vi "MegaAwesome_9_11_12a_JW.vi"() -> ()   [LabVIEW 2011]
uses:
  MegaAwesome_States.ctl
  <vilib>/Utility/inputDevices.llb/keyboardAcquire.vi
  <vilib>/Utility/file.llb/Read From Spreadsheet File (string).vi
  <vilib>/Utility/file.llb/Write To Spreadsheet File (string).vi
panel:
  in  "Slider Min":dbl=5.0
  in  "Slider Max":dbl=5.0
  out "Opj X Axis":string
  out "X Axis Display Type":string
  in  "Index-Sat":dbl=5.0
  in  "Index-Lin":dbl=5.0
  in  "IndexLog-Lin":dbl=5.0
  in  "IndexLog-Sat":dbl=5.0 caption="Num Pts"
  out "Lin Id-Log Used":dbl[](array[numeric])
  out "Lin-Vg Array-Log Used":dbl[](array[numeric])
  in  "New: Comments":string
  out "Save Array":string[][](array[string])
  out "Folder Index":i32 caption="Length"
  out "Sat Id-Used":dbl[](array[numeric])
  out "Sat Vg Array-Used":dbl[](array[numeric])
  out "Vg Array-Log-Used":dbl[](array[numeric])
  out "Sat Id-Log-Used":dbl[](array[numeric])
  out "Lin Id-Used":dbl[](array[numeric])
  out "Lin-Vg Array-Used":dbl[](array[numeric])
  out "Lin Vd":dbl
  out "Recorded Prop":T1
  out "Current State":T2
  in  "Main Tab Control":T3(tab)
  in  "Include Images?":bool
  in  "Image Folder":path
  out "Image File":path
  in  "Transfer File":path
  out "Transfer Folder":path
  out "Fabrication Prop":T4
  in  "Include Transport?":bool
  in  "Zoom":i16(slide)=-3 scale=-5.0..5.0
  in  "Magnification":u16(ring) items=["5x", "10x", "20x", "50x", "80x"]
  out "Distances":dbl[](array[numeric])
  in  "Undo Button":bool
  in  "Remove Button":bool
  in  "Transfer Plots":T5(tab)=enum."Saturation"
  in  "Lin-Trans Slider":dbl(slide) step=1.0 scale=-40.0..40.0 scale format="%#_1p"
  out "Sqrt-Lin":cluster{dbl[], dbl[]}[](graph)
  in  "Sat-Trans Slider":dbl(slide) step=1.0 scale=-40.0..40.0 scale format="%#_1p"
  out "Sqrt-Sat":cluster{dbl[], dbl[]}[](graph)
  out "Raw- Lin":cluster{dbl[], dbl[]}[](graph)
  out "Raw- Sat":cluster{dbl[], dbl[]}[](graph)
  in  "Log Plots":enum32{"Linear", "Saturation", "Transport"}(tab)=enum."Saturation"
  in  "Lin-Log Slider":dbl(slide) step=1.0 scale=-40.0..40.0 scale format="%#_1p"
  out "Log-Lin":cluster{dbl[], dbl[]}[](graph)
  in  "Sat-Log Slider":dbl(slide) step=1.0 scale=-40.0..40.0 scale format="%#_1p"
  out "Log-Sat":cluster{dbl[], dbl[]}[](graph)
  out "Transport":cluster{dbl[], dbl[]}[](graph)
  in  "Manual Controls":T6
  in  "File Controls":T7
  out "Date Recorded":string="Date Recorded" caption="Measured"
  out "Data Name:":string
  out "Image Name":string
  out "Index":string
  out "Date Created":string caption="Fabricated"
  in  "Comments:":string
  out "Rec: Length":dbl caption="Length" format="%#_3g"
  out "Rec: Width":dbl caption="Width" format="%#_4g"
  out "Rec: Dielectric (d)":dbl caption="Dielectric (d)" format="%#_3g"
  in  "New: Dielectric":dbl
  in  "New: Length":dbl
  in  "New: Width":dbl
  out "Rec: Temp":dbl caption="Sample Temp" format="%.1f"
  in  "New: Temp":dbl format="%.1f"
  out "Image Out":T8(plugin-control)
  in  "Num Pts":dbl=5.0
  in  "Num Pts Log":dbl=5.0 caption="Num Pts"
  out "Recorded Values Cluster":T9
  out "Calculated Values Cluster":T9 caption="Recorded Values Cluster"
  out "Re-Calculated Values Cluster":T9 caption="Recorded Values Cluster"
  in  "Independant Variable:":string(combo)="Length (um):"
  out "Image Preview":T8(plugin-control)
  out "Total Width":dbl
  in  "No Image File":path=path "\\\\acad1\\physics/Jurchescu-group/JW-PD/Mega Awesome/Image Not Found.png"
  in  "Room Temp":dbl=294.0
  in  "Origin Project File":path=path "\\\\acad1\\physics/Jurchescu-group/JW-PD/Group Library/Origin Project Files/DeviceData_8_10_12a_JW.opj"
  in  "Transport Style Controls":T10={"Transport Line Size"=1, "Transport Line Color"=16772608} {"Transport Line Size" items=["Extra Small", "Small", "Medium", "Large", "Extra Large"]}
  # "Image Location"
  # "(May not work with older versions)"
  # "Recorded"
  # "Calculated"
  # "Re-Calculated"
  # "Manual"
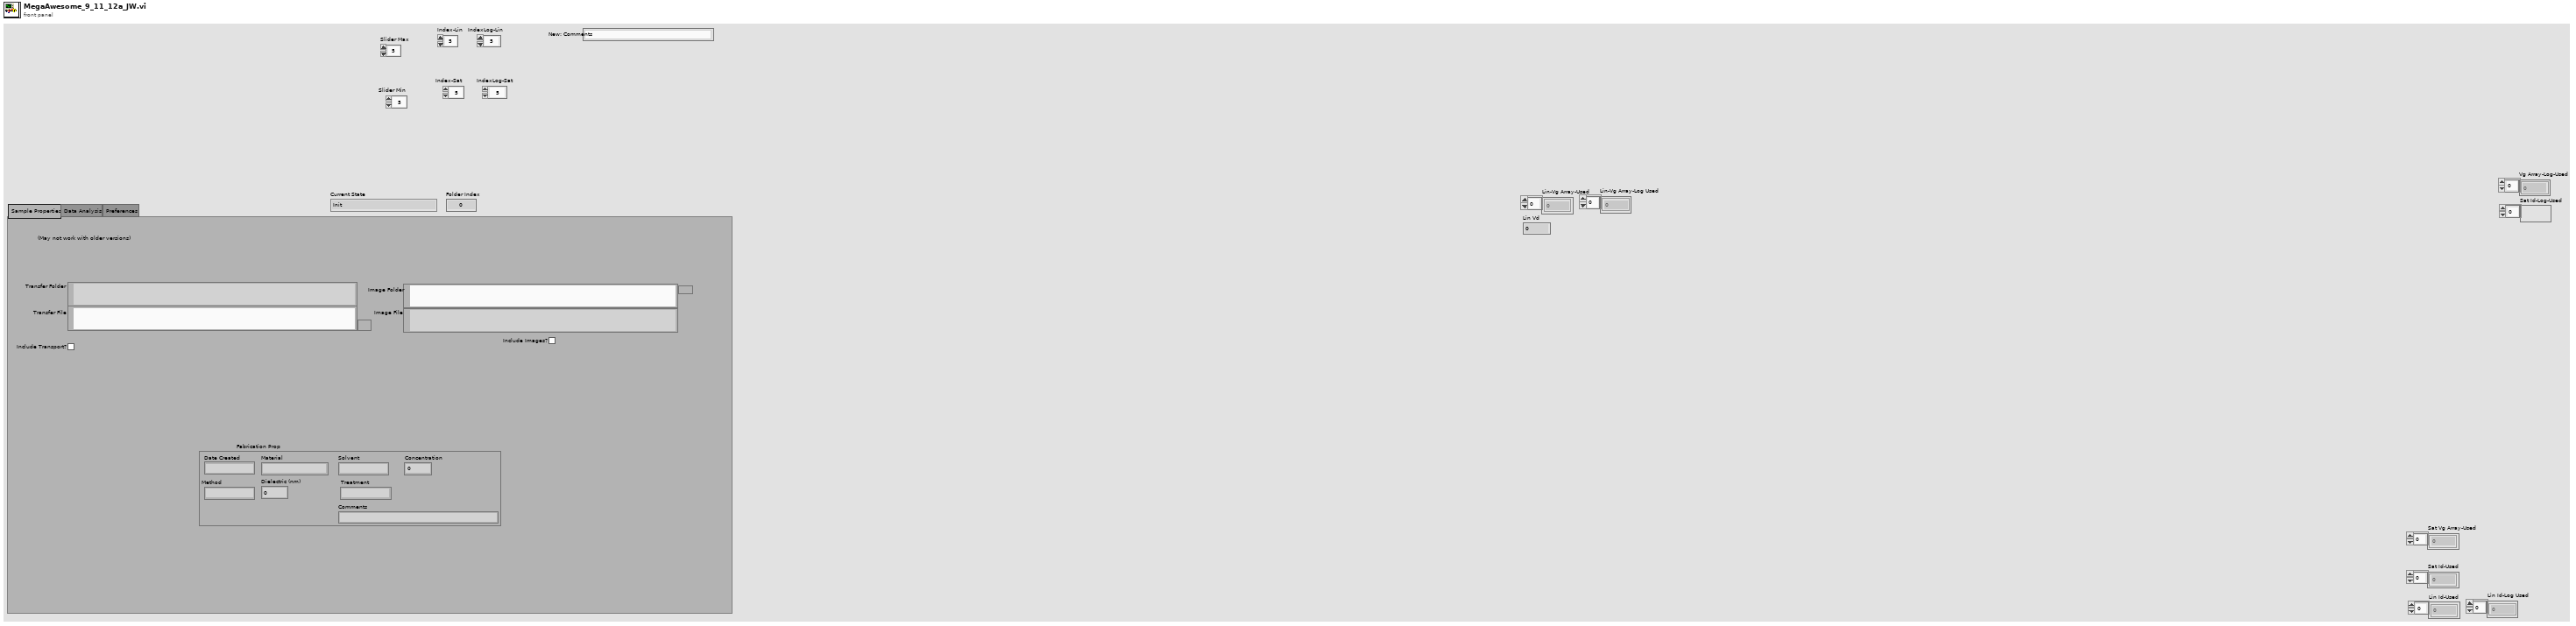
[diagram p1: front panel]
types:
  T1 = cluster{"Date Recorded":string, "Index":string, "Length":dbl, "Width":dbl, "Sample Temp":dbl}
  T2 = typedef "MegaAwesome_States.ctl" = enum16{"Init", "File Missing", "No Event", "Read Data", "Calculated Values", "Re-Calculated Values", "Next File", "Previous File", "Discard File", "Save", "Save Lines", "Export", "Exit"}
  T3 = enum32{"Sample Properties", "Data Analysis", "Preferences"}
  T4 = cluster{"Date Created":string, "Material":string, "Solvent":string, "Concentration":dbl, "Method":string, "Dielectric (nm)":dbl, "Treatment":string, "Comments":string}
  T5 = enum32{"Linear", "Saturation", "Raw-Linear", "Raw-Saturation"}
  T6 = cluster{"Manual-Temp":bool, "Manual-Width":bool, "Manuel-Length":bool, "Manuel-Dielectric":bool, "Manual Comments":bool}
  T7 = cluster{"Previous File":bool, "Discard ":bool, "Save Lines":bool, "Close":bool, "Next File ":bool, "Save":bool, "Save Next":bool, "Export":bool}
  T8 = typedef "IMAQ Image.ctl" = refnum<image>
  T9 = cluster{"Mobility-Sat":dbl, "Moblitity-Lin":dbl, "On/Off":dbl, "Off Current":dbl, "Vt-Sat":dbl, "STS":dbl, "Trap Density-VT":dbl, "Trap Density-STS":dbl}
  T10 = cluster{"Transport Line Size":u16, "Transport Line Color":u32}
  T11 = typedef "LVBoundsTypeDef.ctl" = cluster{"Width":u32, "Height":u32}
  T12 = cluster{"Global Rectangle":i32[], "Contours":cluster{"Contour Type":u32, "ROI Type":u32, "Points":i32[]}[]}
  T13 = cluster{"Contour Type":u32, "ROI Type":u32, "Points":i32[]}[]
  T14 = cluster{i32[], cluster{"Contour Type":u32, "ROI Type":u32, "Points":i32[]}[]}
  T15 = enum16{"0", "1", "2", "3", "4", "5", "6", "7", "8", "9", "A", "B", "C", "D", "E", "F", "G", "H", "I", "J", "K", "L", "M", "N", "O", "P", "Q", "R", "S", "T", "U", "V", "W", "X", "Y", "Z", "F1", "F2", "F3", "F4", "F5", "F6", "F7", "F8", "F9", "F10", "F11", "F12", "F13", "F14", "F15", "ADD", "BACK", "BACKSLASH", "CAPITAL", "COMMA", "DECIMAL", "DELETE", "DIVIDE", "DOWN", "END", "EQUALS", "ESCAPE", "GRAVE (`)", "HOME", "INSERT", "LBRACKET", "LCONTROL", "LEFT", "L ALT", "LSHIFT", "LWIN", "MINUS", "MULTIPLY", "NEXT", "NUMLOCK", "NUMPAD_0", "NUMPAD_1", "NUMPAD_2", "NUMPAD_3", "NUMPAD_4", "NUMPAD_5", "NUMPAD_6", "NUMPAD_7", "NUMPAD_8", "NUMPAD_9", "PAUSE", "PERIOD", "PRIOR (PG UP)", "RBRACKET", "RCONTROL", "RETURN", "RIGHT", "R ALT", "RSHIFT", "RWIN", "SCROLL", "SEMICOLON", "SLASH", "SPACE", "SUBTRACT", "TAB", "UP", "ENTER (num pad)", "' (quote)"}[]
  T16 = enum16{"0", "1", "2", "3", "4", "5", "6", "7", "8", "9", "A", "B", "C", "D", "E", "F", "G", "H", "I", "J", "K", "L", "M", "N", "O", "P", "Q", "R", "S", "T", "U", "V", "W", "X", "Y", "Z", "F1", "F2", "F3", "F4", "F5", "F6", "F7", "F8", "F9", "F10", "F11", "F12", "F13", "F14", "F15", "ADD", "BACK", "BACKSLASH", "CAPITAL", "COMMA", "DECIMAL", "DELETE", "DIVIDE", "DOWN", "END", "EQUALS", "ESCAPE", "GRAVE (`)", "HOME", "INSERT", "LBRACKET", "LCONTROL", "LEFT", "L ALT", "LSHIFT", "LWIN", "MINUS", "MULTIPLY", "NEXT", "NUMLOCK", "NUMPAD_0", "NUMPAD_1", "NUMPAD_2", "NUMPAD_3", "NUMPAD_4", "NUMPAD_5", "NUMPAD_6", "NUMPAD_7", "NUMPAD_8", "NUMPAD_9", "PAUSE", "PERIOD", "PRIOR (PG UP)", "RBRACKET", "RCONTROL", "RETURN", "RIGHT", "R ALT", "RSHIFT", "RWIN", "SCROLL", "SEMICOLON", "SLASH", "SPACE", "SUBTRACT", "TAB", "UP", "ENTER (num pad)", "' (quote)"}
  T17 = typedef "ROI Descriptor" = cluster{"Global Rectangle":i32[], "Contours":cluster{"ID":enum32{"External", "Internal"}, "Type":u32, "Coordinates":i32[]}[]}
  T18 = cluster{string, sgl, bool, bool, bool, bool, bool, bool, i32}
  T19 = cluster{i32, cluster{string, sgl, bool, bool, bool, bool, bool, bool, i32}, i32, i32}
  T20 = cluster{"Contour Type":u32, "ROI Type":u32, "Points":i32[]}
  T21 = cluster{"Points[0]":i32, "Points[1]":i32, "Points[2]":i32, "Points[3]":i32, "Points[4]":i32, "Points[5]":i32, "Points[6]":i32, "Points[7]":i32, "Points[8]":i32}
  T22 = cluster{"[0]":cluster{dbl[], dbl[]}, "[1]":cluster{dbl[], dbl[]}, "[2]":cluster{dbl[], dbl[]}, "[3]":cluster{dbl[], dbl[]}, "[4]":cluster{dbl[], dbl[]}, "[5]":cluster{dbl[], dbl[]}, "[6]":cluster{dbl[], dbl[]}, "[7]":cluster{dbl[], dbl[]}, "[8]":cluster{dbl[], dbl[]}}
  T23 = cluster{"Sat Vg Used":dbl[], "Sat Sqrt(Id) Used ":dbl[], "Lin Vg Used":dbl[], "Lin Sqrt(Id) Used":dbl[], "Index-Lin":dbl, "Index-Sat":dbl}
  T24 = cluster{"Raw Sat":cluster{dbl[], dbl[]}[], "Sqrt Sat":cluster{dbl[], dbl[]}[], "Log Sat":cluster{dbl[], dbl[]}[], "Raw Lin":cluster{dbl[], dbl[]}[], "Sqrt Lin":cluster{dbl[], dbl[]}[], "Log Lin":cluster{dbl[], dbl[]}[]}
  T25 = cluster{"Mobility-Sat":dbl, "Vt-Sat":dbl, "Mobility-Lin":dbl, "Vt-Lin":dbl, "Off I-Sat":dbl, "On/Off I-Sat":dbl}
  T26 = cluster{"Sat Vg Used":dbl[], "Sat Log(Id) Used":dbl[], "Lin Vg Used":dbl[], "Lin Log(Id) Used":dbl[], "STS Index-Sat":dbl, "STS Index-Lin":dbl}
  T27 = cluster{"Independant  Variable Indicator":string, "Parameter String Indicator":string}
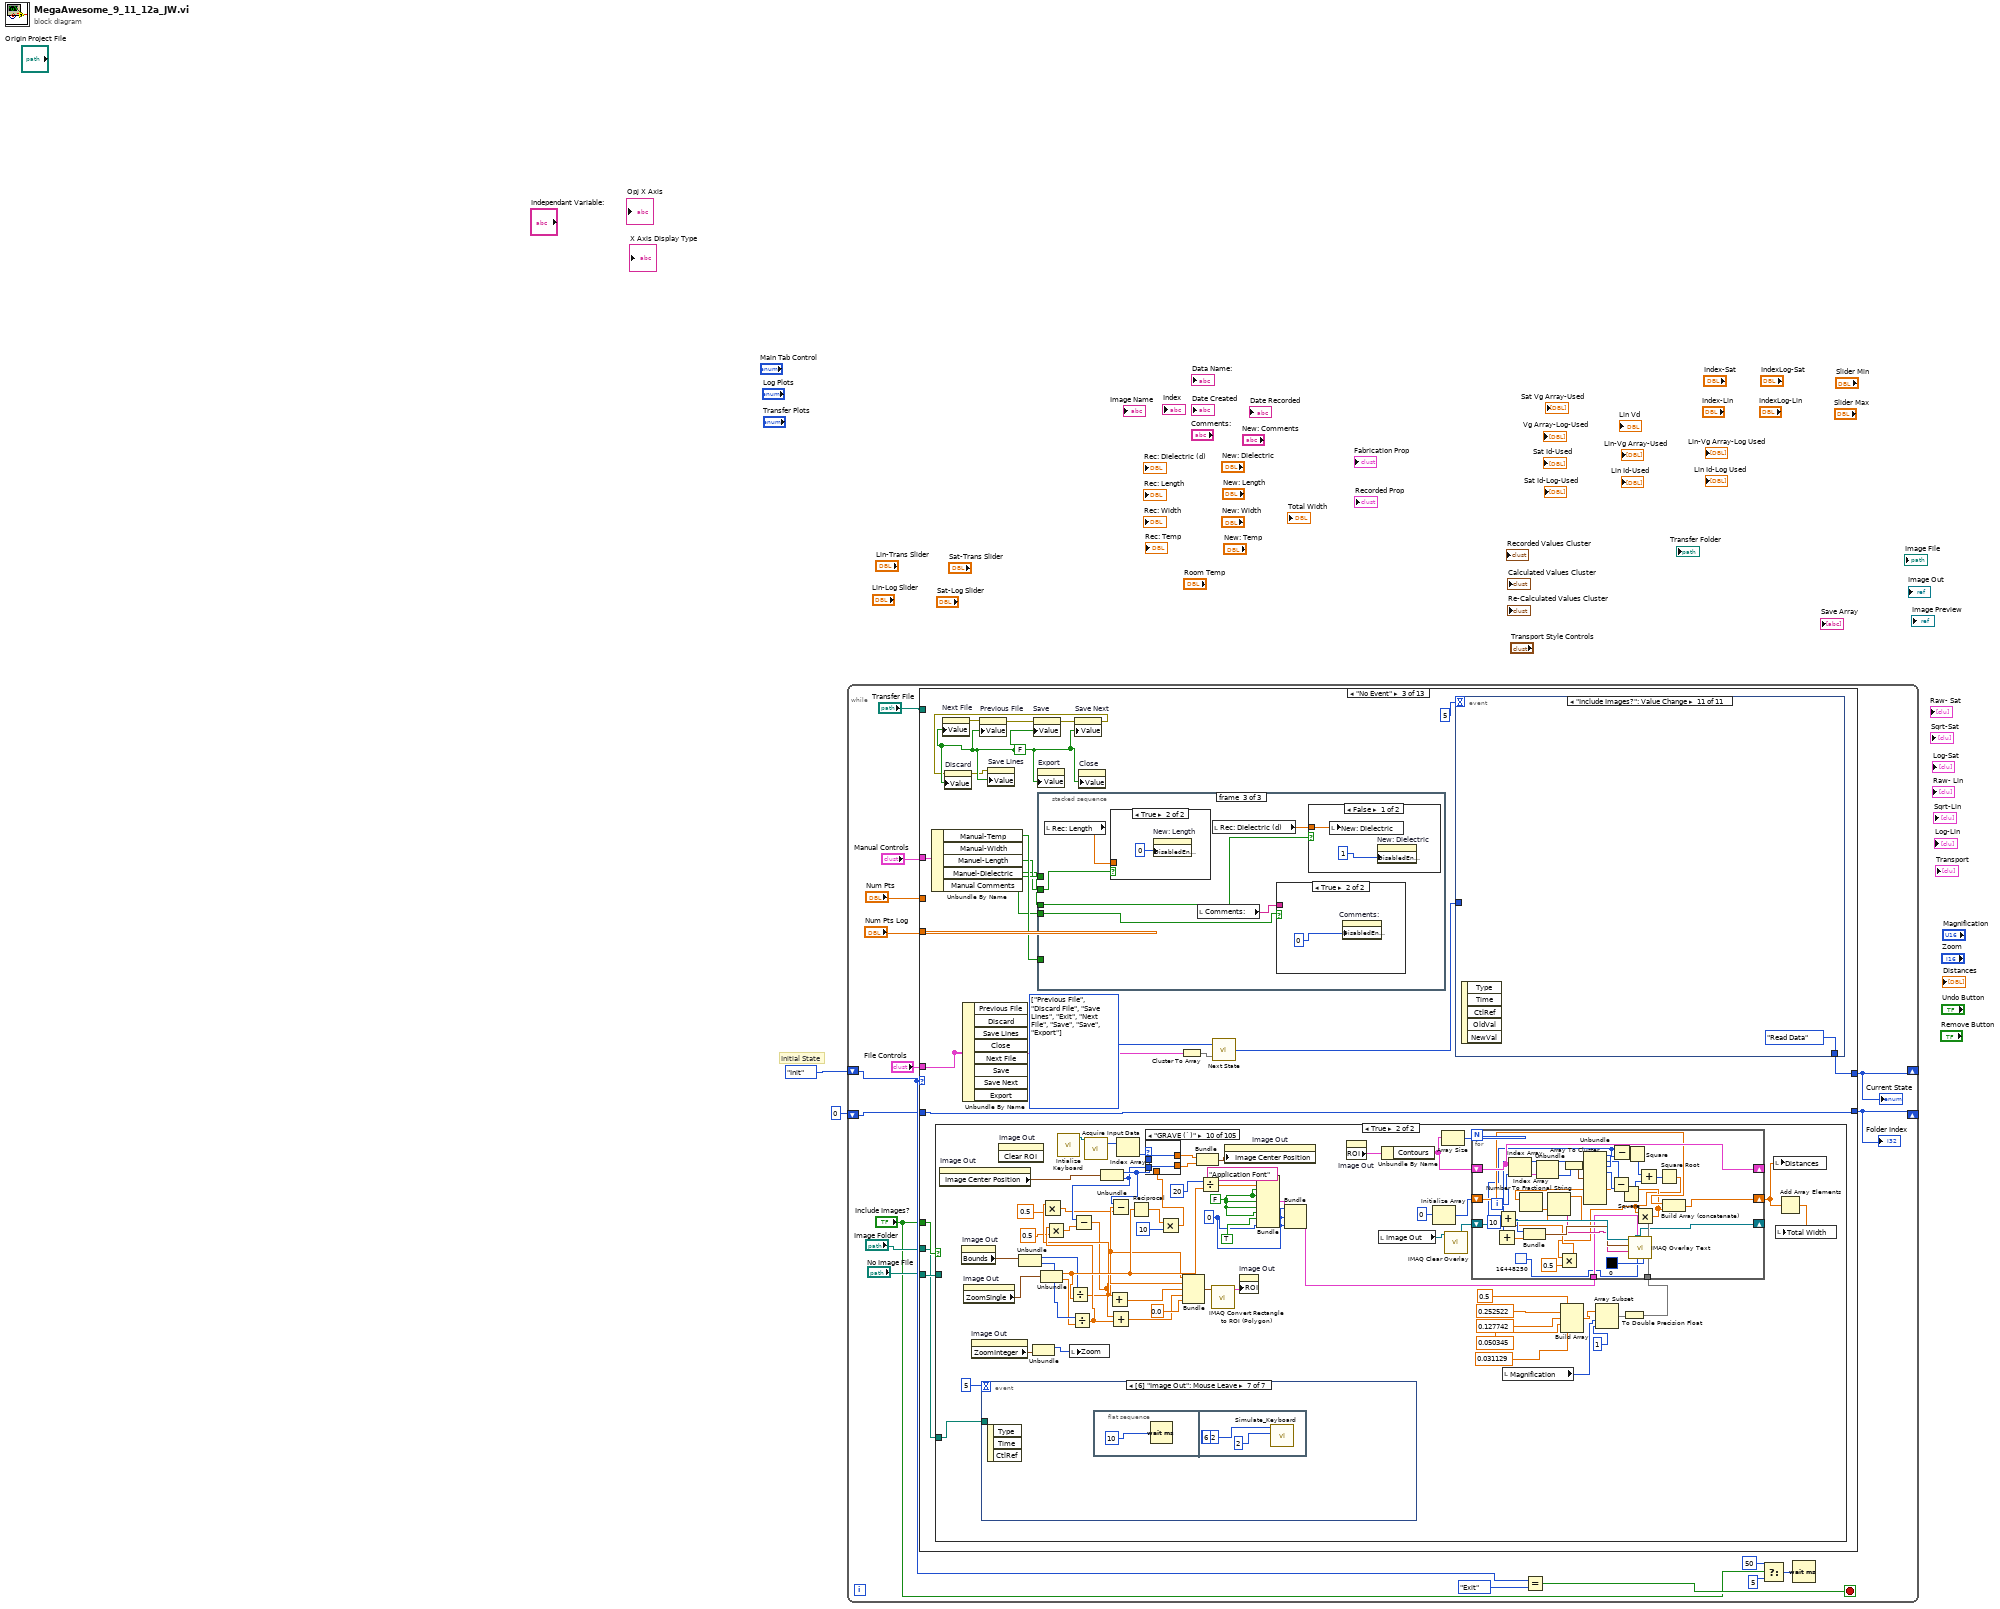
[diagram p0: block diagram]
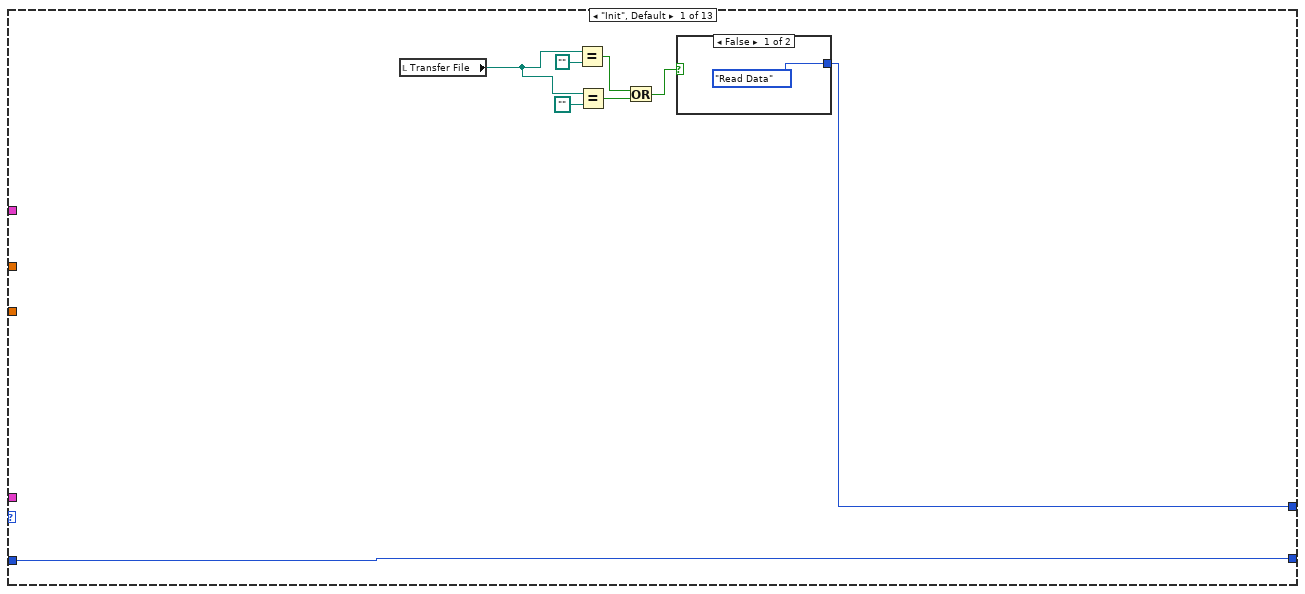
[diagram p2: hidden frame]
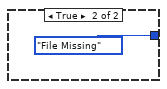
[diagram p3: hidden frame]
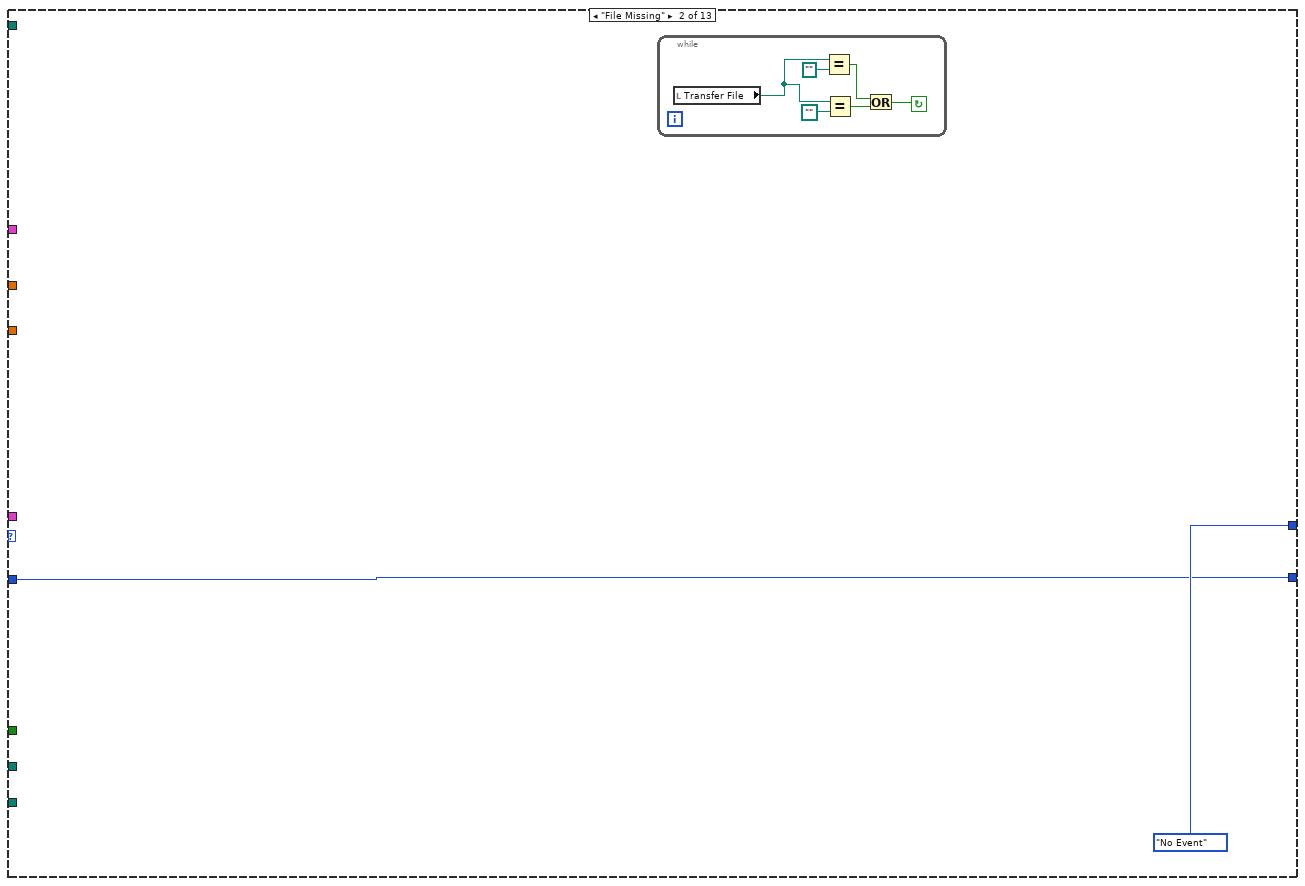
[diagram p4: hidden frame]
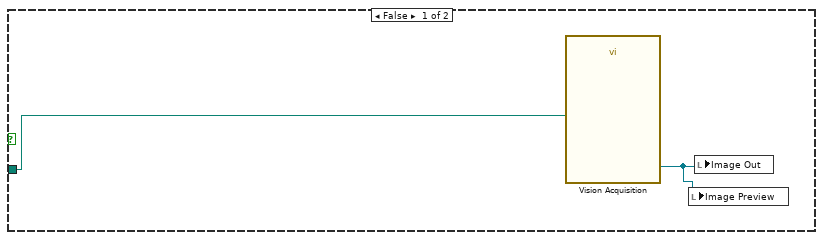
[diagram p5: hidden frame]
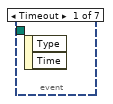
[diagram p6: hidden frame]
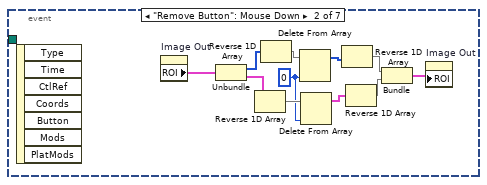
[diagram p7: hidden frame]
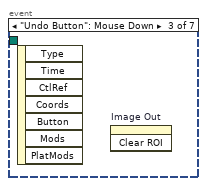
[diagram p8: hidden frame]
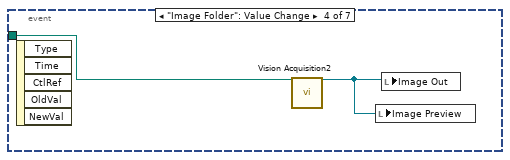
[diagram p9: hidden frame]
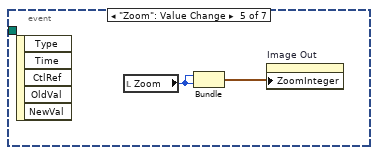
[diagram p10: hidden frame]
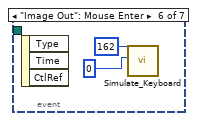
[diagram p11: hidden frame]
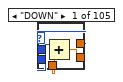
[diagram p12: hidden frame]
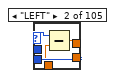
[diagram p13: hidden frame]
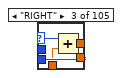
[diagram p14: hidden frame]
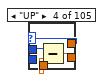
[diagram p15: hidden frame]
diagram:
  # "Initial State"
  n1 = while {
    shift-right: [w16] -> _
    shift-left: MegaAwesome_States."Init" -> [w18]
    shift-right: [w9] -> _
    shift-left: 0 -> [w10]
    stop <- w19 stop-if-true
    n2 = case shown="\"No Event\"" w18 {
      tunnel: [w21 MegaAwesome_States."No Event" w49 MegaAwesome_States."Calculated Values" MegaAwesome_States."Re-Calculated Values" MegaAwesome_States."No Event" MegaAwesome_States."Read Data" MegaAwesome_States."Read Data" MegaAwesome_States."No Event" w688 MegaAwesome_States."No Event" MegaAwesome_States."No Event" MegaAwesome_States."Exit"] -> w16
      tunnel: "Transfer File" -> [_ _ _ w529 w561 _ w657 w669 _ w693 _ _ _]
      tunnel: "Num Pts" -> [_ _ _ _ w585 _ _ _ _ _ _ _ _]
      tunnel: "Num Pts Log" -> [_ _ _ _ w584 _ _ _ _ _ _ _ _]
      tunnel: "Image Folder" -> [_ _ w38 _ w581 _ _ _ _ _ _ w1213 _]
      tunnel: "No Image File" -> [_ _ w39 _ w580 _ _ _ _ _ _ _ _]
      tunnel: [w20 w30 w57 w523 w579 w617 w642 w667 w685 w694 w1209 w1222 w1226] -> w9
      tunnel: w10 -> [w20 w30 w57 _ w579 w617 w643 w668 w685 w694 w1209 w1222 w1226]
      tunnel: "Manual Controls" -> [_ _ w51 _ _ _ _ _ _ w692 _ _ _]
      tunnel: "File Controls" -> [_ _ w47 _ _ _ _ _ _ w687 _ _ _]
      tunnel: "Include Images?" -> [_ _ w40 _ w550 _ _ _ _ _ _ _ _]
      frame "Init", Default {
        n3 = local read "Transfer File"() -> (w22:path)
        n4 = Equal?(x=w22, y=path "") -> (x = y?=w25:bool)
        n5 = Equal?(x=w22, y=path "") -> (x = y?=w24:bool)
        n6 = Or(x=w25, y=w24) -> (x .or. y?=w27:bool)
        n7 = case shown="False" w27 {
          tunnel: [MegaAwesome_States."Read Data" MegaAwesome_States."File Missing"] -> w21
          frame False {
          }
          frame True {
          }
        }
      }
      frame "File Missing" {
        n8 = while {
          stop <- w32 continue-if-true
          n9 = local read "Transfer File"() -> (w33:path)
          n10 = Equal?(x=w33, y=path "") -> (x = y?=w35:bool)
          n11 = Equal?(x=w33, y=path "") -> (x = y?=w36:bool)
          n12 = Or(x=w35, y=w36) -> (x .or. y?=w32:bool)
        }
      }
      frame "No Event" {
        w46 = FALSE
        w59 = T2[] [enum."Previous File", enum."Discard File", enum."Save Lines", enum."Exit", enum."Next File", enum."Save", enum."Save", enum."Export"] items=["Init", "File Missing", "No Event", "Read Data", "Calculated Values", "Re-Calculated Values", "Next File", "Previous File", "Discard File", "Save", "Save Lines", "Export", "Exit"]
        n13 = Unbundle By Name(w51) -> ("Manual-Temp"=w56:bool, "Manual-Width"=w55:bool, "Manuel-Length"=w54:bool, "Manuel-Dielectric"=w53:bool, "Manual Comments"=w52:bool)
        n14 = case shown="True" w40 {
          tunnel: w39 -> [w60 _]
          tunnel: w38 -> [_ w62]
          frame False {
            n15 = call "Vision Acquisition"("Image Path"=w60) -> ("Image Out"=w61:T8)  [unwired: 25 in, 1 out]
            n16 = local write "Image Preview"(w61) -> ()
            n17 = local write "Image Out"(w61) -> ()
          }
          frame True {
            w114 = FALSE
            w116 = 0
            n18 = property on="Image Out" class="ImageControl"() -> ("Image Center Position"=w86:cluster{"X":u32, "Y":u32})  [unwired: 2 in, 2 out]
            n19 = property on="Image Out" class="ImageControl"() -> ("Bounds"=w87:T11)  [unwired: 2 in, 2 out]
            n20 = property on="Image Out" class="ImageControl"() -> ("ZoomSingle"=w88:cluster{"X":sgl, "Y":sgl})  [unwired: 2 in, 2 out]
            n21 = property on="Image Out" class="ImageControl"() -> ("ZoomInteger"=w89:cluster{"X":i32, "Y":i32})  [unwired: 2 in, 2 out]
            n22 = event shown="[6] \"Image Out\": Mouse Leave" {
              selector: _ -> [_ _ _ _ _ _ _]
              dyn-events: _ -> [_ _ _ _ _ _ _]
              timeout: 5 -> [_ _ _ _ _ _ _]
              tunnel: w62 -> [_ _ _ w136 _ _ _]
              event Timeout {
                n23 = event-data() -> ()  [unwired: 1 in, 2 out]
              }
              event "Remove Button": Mouse Down {
                w124 = 0
                n24 = event-data() -> ()  [unwired: 1 in, 7 out]
                n25 = property on="Image Out" class="ImageControl"() -> ("ROI"=w126:T12)  [unwired: 2 in, 2 out]
                n26 = Unbundle(w126) -> ("Global Rectangle"=w134:i32[], "Contours"=w132:T13)
                n27 = Reverse 1D Array(array=w132) -> (reversed array=w131:T13)
                n28 = Reverse 1D Array(array=w134) -> (reversed array=w133:i32[])
                n29 = Delete From Array(array=w133, index=w124) -> (array with subset deleted=w130:i32[])  [unwired: 1 in, 1 out]
                n30 = Delete From Array(array=w131, index=w124) -> (array with subset deleted=w129:T13)  [unwired: 1 in, 1 out]
                n31 = Reverse 1D Array(array=w130) -> (reversed array=w128:i32[])
                n32 = Reverse 1D Array(array=w129) -> (reversed array=w127:T13)
                n33 = Bundle(w128, w127) -> (w125:T14)  [unwired: 1 in]
                n34 = property on="Image Out" class="ImageControl"("ROI"=w125) -> ()  [unwired: 2 in, 2 out]
              }
              event "Undo Button": Mouse Down {
                n35 = event-data() -> ()  [unwired: 1 in, 7 out]
                n36 = invoke on="Image Out" class="ImageControl" method="Clear ROI"() -> ()  [unwired: 3 in, 3 out]
              }
              event "Image Folder": Value Change {
                n37 = event-data() -> ()  [unwired: 1 in, 5 out]
                n38 = call "Vision Acquisition2"("Image Path"=w136) -> ("Image Out"=w135:T8)  [unwired: 25 in, 1 out]
                n39 = local write "Image Preview"(w135) -> ()
                n40 = local write "Image Out"(w135) -> ()
              }
              event "Zoom": Value Change {
                n41 = event-data() -> ()  [unwired: 1 in, 5 out]
                n42 = local read "Zoom"() -> (w138:i16)
                n43 = Bundle("Zoom"=w138, "Zoom"=w138) -> (w137:cluster{"Zoom":i16, "Zoom":i16})  [unwired: 1 in]
                n44 = property on="Image Out" class="ImageControl"("ZoomInteger"=w137) -> ()  [unwired: 2 in, 2 out]
              }
              event "Image Out": Mouse Enter {
                n45 = event-data() -> ()  [unwired: 1 in, 3 out]
                n46 = call "Simulate_Keyboard.vi"("Action"=0, "Virtual Key"=162) -> ()  [unwired: 7 in, 1 out]
              }
              event "Image Out": Mouse Leave {
                n47 = event-data() -> ()  [unwired: 1 in, 3 out]
                n48 = flat-sequence {
                  frame #0 {
                    n49 = Wait (ms)(milliseconds to wait=10) -> ()  [unwired: 1 out]
                  }
                  frame #1 {
                    (unwired) 6
                    n50 = call "Simulate_Keyboard.vi"("Action"=2, "Virtual Key"=162) -> ()  [unwired: 7 in, 1 out]
                  }
                }
              }
            }
            n51 = invoke on="Image Out" class="ImageControl" method="Clear ROI"() -> ()  [unwired: 3 in, 3 out]
            n52 = Unbundle(w87) -> ("Width"=w101:u32, "Height"=w102:u32)
            n53 = Unbundle(w89) -> ("X"=w90:i32)  [unwired: 1 out]
            n54 = Unbundle(w88) -> ("X"=w121:sgl, "Y"=w100:sgl)
            n55 = call <vilib>:"Intialize Keyboard.vi"() -> ("device ID"=w94:refnum<k1>)  [unwired: 10 in, 1 out]
            n56 = Divide(x=w101, y=w121) -> (x/y=w111:sgl)
            n57 = Multiply(x=w111, y=0.5) -> (x*y=w105:dbl)
            n58 = local write "Zoom"(w90) -> ()
            n59 = Divide(x=w102, y=w100) -> (x/y=w112:sgl)
            n60 = Multiply(x=w112, y=0.5) -> (x*y=w106:dbl)
            n61 = call-poly <vilib>:"Acquire Input Data.vi"("device ID"=w94) -> ("keys pressed"=w95:T15)  [unwired: 16 in, 2 out]
            n62 = Unbundle(w86) -> ("X"=w110:u32, "Y"=w109:u32)
            n63 = Subtract(x=w109, y=w106) -> (x-y=w108:dbl)
            n64 = Subtract(x=w110, y=w105) -> (x-y=w107:dbl)
            n65 = Add(x=w107, y=w111) -> (x+y=w96:dbl)
            n66 = Add(x=w108, y=w112) -> (x+y=w97:dbl)
            n67 = Index Array(array=w95) -> (element=w91:T16)  [unwired: 1 in]
            n68 = Reciprocal(x=w121) -> (1/x=w122:sgl)
            n69 = Multiply(x=w122, y=10) -> (x*y=w120:sgl)
            n70 = case shown="\"GRAVE (`)\"" w91 {
              tunnel: w110 -> [w145 w151 w155 w157 w161 w163 w165 w167 w169 w171 w173 w175 w177 w179 w181 w183 w185 w187 w189 w191 w193 w195 w197 w199 w201 w203 w205 w207 w209 w211 w213 w215 w217 w219 w221 w223 w225 w227 w229 w231 w233 w235 w237 w239 w241 w243 w245 w247 w249 w251 w253 w255 w257 w259 w261 w263 w265 w267 w269 w271 w273 w275 w277 w279 w281 w283 w285 w287 w289 w291 w293 w295 w297 w299 w301 w303 w305 w307 w309 w311 w313 w315 w317 w319 w321 w323 w325 w327 w329 w331 w333 w335 w337 w339 w341 w343 w345 w347 w349 w351 w353 w355 w357 w359 w361]
              tunnel: [w145 w150 w154 w157 w161 w163 w165 w167 w169 w171 w173 w175 w177 w179 w181 w183 w185 w187 w189 w191 w193 w195 w197 w199 w201 w203 w205 w207 w209 w211 w213 w215 w217 w219 w221 w223 w225 w227 w229 w231 w233 w235 w237 w239 w241 w243 w245 w247 w249 w251 w253 w255 w257 w259 w261 w263 w265 w267 w269 w271 w273 w275 w277 w279 w281 w283 w285 w287 w289 w291 w293 w295 w297 w299 w301 w303 w305 w307 w309 w311 w313 w315 w317 w319 w321 w323 w325 w327 w329 w331 w333 w335 w337 w339 w341 w343 w345 w347 w349 w351 w353 w355 w357 w359 w361] -> w92
              tunnel: w109 -> [w147 w149 w153 w159 w160 w162 w164 w166 w168 w170 w172 w174 w176 w178 w180 w182 w184 w186 w188 w190 w192 w194 w196 w198 w200 w202 w204 w206 w208 w210 w212 w214 w216 w218 w220 w222 w224 w226 w228 w230 w232 w234 w236 w238 w240 w242 w244 w246 w248 w250 w252 w254 w256 w258 w260 w262 w264 w266 w268 w270 w272 w274 w276 w278 w280 w282 w284 w286 w288 w290 w292 w294 w296 w298 w300 w302 w304 w306 w308 w310 w312 w314 w316 w318 w320 w322 w324 w326 w328 w330 w332 w334 w336 w338 w340 w342 w344 w346 w348 w350 w352 w354 w356 w358 w360]
              tunnel: [w146 w149 w153 w158 w160 w162 w164 w166 w168 w170 w172 w174 w176 w178 w180 w182 w184 w186 w188 w190 w192 w194 w196 w198 w200 w202 w204 w206 w208 w210 w212 w214 w216 w218 w220 w222 w224 w226 w228 w230 w232 w234 w236 w238 w240 w242 w244 w246 w248 w250 w252 w254 w256 w258 w260 w262 w264 w266 w268 w270 w272 w274 w276 w278 w280 w282 w284 w286 w288 w290 w292 w294 w296 w298 w300 w302 w304 w306 w308 w310 w312 w314 w316 w318 w320 w322 w324 w326 w328 w330 w332 w334 w336 w338 w340 w342 w344 w346 w348 w350 w352 w354 w356 w358 w360] -> w93
              tunnel: w120 -> [w144 w148 w152 w156 _ _ _ _ _ _ _ _ _ _ _ _ _ _ _ _ _ _ _ _ _ _ _ _ _ _ _ _ _ _ _ _ _ _ _ _ _ _ _ _ _ _ _ _ _ _ _ _ _ _ _ _ _ _ _ _ _ _ _ _ _ _ _ _ _ _ _ _ _ _ _ _ _ _ _ _ _ _ _ _ _ _ _ _ _ _ _ _ _ _ _ _ _ _ _ _ _ _ _ _ _]
              frame "DOWN" {
                n71 = Add(x=w147, y=w144) -> (x+y=w146:sgl)
              }
              frame "LEFT" {
                n72 = Subtract(x=w151, y=w148) -> (x-y=w150:sgl)
              }
              frame "RIGHT" {
                n73 = Add(x=w155, y=w152) -> (x+y=w154:sgl)
              }
              frame "UP" {
                n74 = Subtract(x=w159, y=w156) -> (x-y=w158:sgl)
              }
              frame "ENTER (num pad)" {
              }
              frame "' (quote)" {
              }
              frame "END" {
              }
              frame "EQUALS" {
              }
              frame "ESCAPE" {
              }
              frame "GRAVE (`)" {
              }
              frame "HOME" {
              }
              frame "INSERT" {
              }
              frame "LBRACKET" {
              }
              frame "LCONTROL" {
              }
              frame "L ALT" {
              }
              frame "LSHIFT" {
              }
              frame "LWIN" {
              }
              frame "MINUS" {
              }
              frame "MULTIPLY" {
              }
              frame "NEXT" {
              }
              frame "NUMLOCK" {
              }
              frame "NUMPAD_0" {
              }
              frame "NUMPAD_1" {
              }
              frame "NUMPAD_2" {
              }
              frame "NUMPAD_3" {
              }
              frame "NUMPAD_4" {
              }
              frame "NUMPAD_5" {
              }
              frame "NUMPAD_6" {
              }
              frame "NUMPAD_7" {
              }
              frame "NUMPAD_8" {
              }
              frame "NUMPAD_9" {
              }
              frame "PAUSE" {
              }
              frame "PERIOD" {
              }
              frame "PRIOR (PG UP)" {
              }
              frame "RBRACKET" {
              }
              frame "RCONTROL" {
              }
              frame "RETURN" {
              }
              frame "R ALT" {
              }
              frame "RSHIFT" {
              }
              frame "RWIN" {
              }
              frame "SCROLL" {
              }
              frame "SEMICOLON" {
              }
              frame "SLASH" {
              }
              frame "SPACE" {
              }
              frame "SUBTRACT" {
              }
              frame "TAB" {
              }
              frame "DIVIDE" {
              }
              frame "DELETE" {
              }
              frame "DECIMAL" {
              }
              frame "COMMA" {
              }
              frame "CAPITAL" {
              }
              frame "BACKSLASH" {
              }
              frame "BACK" {
              }
              frame "ADD" {
              }
              frame "F15" {
              }
              frame "F14" {
              }
              frame "F13" {
              }
              frame "F12" {
              }
              frame "F11" {
              }
              frame "F10" {
              }
              frame "F9" {
              }
              frame "F8" {
              }
              frame "F7" {
              }
              frame "F6" {
              }
              frame "F5" {
              }
              frame "F4" {
              }
              frame "F3" {
              }
              frame "F2" {
              }
              frame "F1" {
              }
              frame "Z" {
              }
              frame "Y" {
              }
              frame "X" {
              }
              frame "W" {
              }
              frame "V" {
              }
              frame "U" {
              }
              frame "T" {
              }
              frame "S" {
              }
              frame "R" {
              }
              frame "Q" {
              }
              frame "P" {
              }
              frame "O" {
              }
              frame "N" {
              }
              frame "M" {
              }
              frame "L" {
              }
              frame "K" {
              }
              frame "J" {
              }
              frame "I" {
              }
              frame "H" {
              }
              frame "G" {
              }
              frame "F" {
              }
              frame "E" {
              }
              frame "D" {
              }
              frame "C" {
              }
              frame "B" {
              }
              frame "A" {
              }
              frame "9" {
              }
              frame "8" {
              }
              frame "7" {
              }
              frame "6" {
              }
              frame "5" {
              }
              frame "4" {
              }
              frame "3" {
              }
              frame "2" {
              }
              frame "1" {
              }
              frame "0" {
              }
            }
            n75 = Bundle(w107, w108, w96, w97, 0.0) -> (w98:cluster{dbl, dbl, dbl, dbl, dbl})  [unwired: 1 in]
            n76 = Bundle("X"=w92, "Y"=w93) -> (w85:cluster{"X":sgl, "Y":sgl})  [unwired: 1 in]
            n77 = Divide(x=20, y=w121) -> (x/y=w118:sgl)
            n78 = call "IMAQ Convert Rectangle to ROI (Polygon)"("Rectangle"=w98) -> ("ROI Descriptor"=w84:T17)  [unwired: 7 in, 2 out]
            n79 = property on="Image Out" class="ImageControl"("Image Center Position"=w85) -> ()  [unwired: 2 in, 2 out]
            n80 = property on="Image Out" class="ImageControl"("ROI"=w84) -> ()  [unwired: 2 in, 2 out]
            n81 = Bundle("Application Font", w118, w114, w114, w114, w114, w114, TRUE, w116) -> (w113:T18)  [unwired: 1 in]
            n82 = Bundle(w116, w113, w116, w116) -> (w65:T19)  [unwired: 1 in]
            n83 = property on="Image Out" class="ImageControl"() -> ("ROI"=w64:T12)  [unwired: 2 in, 2 out]
            n84 = local read "Image Out"() -> (w66:T8)
            n85 = Unbundle By Name(w64) -> ("Contours"=w70:T13)
            n86 = Initialize Array(0) -> (w72:i32[])  [unwired: 1 in]
            n87 = Array Size(array=w70) -> (size(s)=w71:i32)
            n88 = call "IMAQ Clear Overlay"("Image"=w66) -> ("Image Out"=w81:T8)  [unwired: 9 in, 1 out]
            n89 = local read "Magnification"() -> (w67:u16)
            n90 = Build Array(0.5, 0.252522, 0.127742, 0.050345, 0.031129) -> (w77:dbl[])
            n91 = Array Subset(array=w77, index=w67, length=1) -> (w79:dbl[])
            n92 = To Double Precision Float(number=w79) -> (double precision float=w80:dbl[])
            n93 = for {
              N: w71 -> [_]
              shift-right: [w384] -> _
              shift-left: w70 -> [w384]
              shift-right: [w382] -> w68
              shift-left: w72 -> [w381]
              tunnel: w80 -> [w380]
              shift-right: [w377] -> _
              shift-left: w81 -> [w379]
              tunnel: w65 -> [w372]
              i -> [w376]
              n94 = Index Array(array=w384, index=w376) -> (element=w393:T20)
              n95 = Unbundle(w393) -> ("Points"=w392:i32[])  [unwired: 2 out]
              n96 = Array To Cluster(array=w392) -> (cluster=w391:T21)
              n97 = Unbundle(w391) -> ("Points[0]"=w371:i32, "Points[1]"=w368:i32, "Points[2]"=w383:i32, "Points[3]"=w389:i32)  [unwired: 5 out]
              n98 = Add(x=w371, y=10) -> (x+y=w369:i32)
              n99 = Subtract(x=w368, y=w389) -> (x-y=w388:i32)
              n100 = Subtract(x=w371, y=w383) -> (x-y=w390:i32)
              n101 = Square(x=w388) -> (x^2=w386:i32)
              n102 = Square(x=w390) -> (x^2=w387:i32)
              n103 = Add(x=w387, y=w386) -> (x+y=w385:i32)
              n104 = Square Root(x=w385) -> (sqrt(x)=w362:dbl)
              n105 = Multiply(x=w362, y=0.5) -> (x*y=w365:dbl)
              n106 = Add(x=w365, y=w368) -> (x+y=w367:dbl)
              n107 = Bundle(w369, w367) -> (w378:cluster{i32, dbl})  [unwired: 1 in]
              n108 = Multiply(x=w362, y=w380) -> (x*y=w375:dbl[])
              n109 = Index Array(array=w375) -> (element=w374:dbl)  [unwired: 1 in]
              n110 = Number To Fractional String(number=w374) -> (F-format string=w373:string)  [unwired: 3 in]
              n111 = call "IMAQ Overlay Text"("BG Color (Transparent)"=u32 0, "Text Color (black)"=u32 16448250, "Font, Size & Style"=w372, "String"=w373, "Origin"=w378, "Image"=w379) -> ("Image Out"=w377:T8)  [unwired: 4 in, 1 out]
              n112 = Build Array (concatenate)(w381, w375) -> (w382:dbl[])
            }
            n113 = local write "Distances"(w68) -> ()
            n114 = Add Array Elements(numeric array=w68) -> (sum=w69:dbl)
            n115 = local write "Total Width"(w69) -> ()
          }
        }
        n116 = property on="Next File" class="Bool (strict)"("Value"=w46) -> (error out=w45:errorcluster)  [unwired: 2 in, 1 out]
        n117 = Unbundle By Name(w47) -> ()  [unwired: 8 out]
        n118 = property on="Previous File" class="Bool (strict)"(error in=w45, "Value"=w46) -> (error out=w44:errorcluster)  [unwired: 1 in, 1 out]
        n119 = property on="Save" class="Bool (strict)"(error in=w44, "Value"=w46) -> (error out=w43:errorcluster)  [unwired: 1 in, 1 out]
        n120 = property on="Export" class="Bool (strict)"("Value"=w46) -> ()  [unwired: 2 in, 2 out]
        n121 = stacked-sequence {
          tunnel: w56 -> [w487 _ _]
          tunnel: w55 -> [_ w497 _]
          tunnel: w54 -> [_ _ w512]
          tunnel: w53 -> [_ _ w509]
          tunnel: w52 -> [_ _ w508]
          frame #0 {
            n122 = local read "Rec: Temp"() -> (w486:dbl)
            n123 = case shown="False" w487 {
              tunnel: w486 -> [w492 _]
              tunnel: [w489 w496] -> _
              frame False {
                n124 = local read "Rec: Temp"() -> (w490:dbl)
                n125 = property on="New: Temp" class="DigNum (strict)"("DisabledEnum"=1) -> ()  [unwired: 2 in, 2 out]
                n126 = Equal To 0?(x=w490) -> (x = 0?=w491:bool)
                n127 = local write "New: Temp"(w492) -> ()
                n128 = case shown="True" w491 {
                  tunnel: [w493 w494] -> w489
                  tunnel: w490 -> [w493 _]
                  frame False {
                  }
                  frame True {
                    n129 = local read "Room Temp"() -> (w494:dbl)
                  }
                }
                n130 = local write "New: Temp"(w489) -> ()
              }
              frame True {
                n131 = property on="New: Temp" class="DigNum (strict)"("DisabledEnum"=0) -> ()  [unwired: 2 in, 2 out]
                n132 = local read "New: Temp"() -> (w496:dbl)
              }
            }
          }
          frame #1 {
            n133 = case shown="False" w497 {
              frame False {
                n134 = property on="New: Width" class="DigNum (strict)"("DisabledEnum"=1) -> ()  [unwired: 2 in, 2 out]
              }
              frame True {
                (unwired) 0
              }
            }
            n135 = local read "Total Width"() -> (w503:dbl)
            n136 = Equal To 0?(x=w503) -> (x = 0?=w500:bool)
            n137 = local read "Rec: Width"() -> (w501:dbl)
            n138 = Not(x=w497) -> (.not. x?=w499:bool)
            n139 = Or(x=w500, y=w497) -> (x .or. y?=w502:bool)
            n140 = And(x=w500, y=w499) -> (x .and. y?=w498:bool)
            n141 = case shown="True" w498 {
              tunnel: w501 -> [_ w505]
              frame False {
              }
              frame True {
                n142 = local write "New: Width"(w505) -> ()
              }
            }
            n143 = case shown="True" w502 {
              tunnel: w503 -> [w506 _]
              frame False {
                (unwired) 1
                n144 = local write "New: Width"(w506) -> ()
              }
              frame True {
                n145 = property on="New: Width" class="DigNum (strict)"("DisabledEnum"=0) -> ()  [unwired: 2 in, 2 out]
              }
            }
          }
          frame #2 {
            n146 = local read "Rec: Length"() -> (w513:dbl)
            n147 = case shown="True" w512 {
              tunnel: w513 -> [w521 _]
              frame False {
                n148 = local write "New: Length"(w521) -> ()
                n149 = property on="New: Length" class="DigNum (strict)"("DisabledEnum"=1) -> ()  [unwired: 2 in, 2 out]
              }
              frame True {
                n150 = property on="New: Length" class="DigNum (strict)"("DisabledEnum"=0) -> ()  [unwired: 2 in, 2 out]
              }
            }
            n151 = local read "Comments:"() -> (w510:string)
            n152 = local read "Rec: Dielectric (d)"() -> (w511:dbl)
            n153 = case shown="True" w508 {
              tunnel: w510 -> [w515 _]
              frame False {
                n154 = local write "New: Comments"(w515) -> ()
                n155 = property on="Comments:" class="Str"("DisabledEnum"=1) -> ()  [unwired: 2 in, 2 out]
              }
              frame True {
                n156 = property on="Comments:" class="Str"("DisabledEnum"=0) -> ()  [unwired: 2 in, 2 out]
              }
            }
            n157 = case shown="False" w509 {
              tunnel: w511 -> [w518 _]
              frame False {
                n158 = local write "New: Dielectric"(w518) -> ()
                n159 = property on="New: Dielectric" class="DigNum (strict)"("DisabledEnum"=1) -> ()  [unwired: 2 in, 2 out]
              }
              frame True {
                n160 = property on="New: Dielectric" class="DigNum (strict)"("DisabledEnum"=0) -> ()  [unwired: 2 in, 2 out]
              }
            }
          }
        }
        n161 = property on="Save Next" class="Bool (strict)"(error in=w43, "Value"=w46) -> (error out=w42:errorcluster)  [unwired: 1 in, 1 out]
        n162 = property on="Discard" class="Bool (strict)"(error in=w42, "Value"=w46) -> (error out=w41:errorcluster)  [unwired: 1 in, 1 out]
        n163 = property on="Save Lines" class="Bool (strict)"(error in=w41, "Value"=w46) -> ()  [unwired: 1 in, 2 out]
        n164 = property on="Close" class="Bool (strict)"("Value"=w46) -> ()  [unwired: 2 in, 2 out]
        n165 = Cluster To Array(cluster=w47) -> (array=w58:bool[])
        n166 = call "Next State.vi"("Buttons []"=w58, "States []"=w59) -> ("Enum"=w50:T2)
        n167 = event shown="[10] \"Include Images?\": Value Change" {
          selector: _ -> [_ _ _ _ _ _ _ _ _ _ _]
          dyn-events: _ -> [_ _ _ _ _ _ _ _ _ _ _]
          timeout: 5 -> [_ _ _ _ _ _ _ _ _ _ _]
          tunnel: w50 -> [w394 _ _ _ _ _ _ _ _ _ _]
          tunnel: [w394 MegaAwesome_States."Re-Calculated Values" MegaAwesome_States."Re-Calculated Values" MegaAwesome_States."Re-Calculated Values" MegaAwesome_States."Re-Calculated Values" MegaAwesome_States."Calculated Values" MegaAwesome_States."Re-Calculated Values" MegaAwesome_States."Re-Calculated Values" MegaAwesome_States."Re-Calculated Values" MegaAwesome_States."Re-Calculated Values" MegaAwesome_States."Read Data"] -> w49
          event Timeout {
            n168 = event-data() -> ()  [unwired: 1 in, 2 out]
          }
          event "New: Dielectric": Value Change {
            n169 = event-data() -> ()  [unwired: 1 in, 5 out]
          }
          event "New: Length": Value Change {
            n170 = event-data() -> ()  [unwired: 1 in, 5 out]
          }
          event "New: Width": Value Change {
            n171 = event-data() -> ()  [unwired: 1 in, 5 out]
          }
          event "New: Temp": Value Change {
            n172 = event-data() -> ()  [unwired: 1 in, 5 out]
          }
          event "Num Pts Log", "Transport Style Controls", "Num Pts": Value Change {
            n173 = event-data() -> ()  [unwired: 1 in, 5 out]
          }
          event "Sat-Trans Slider": Value Change {
            n174 = event-data() -> ()  [unwired: 1 in, 5 out]
            n175 = local read "Sqrt-Sat"() -> (w423:cluster{dbl[], dbl[]}[])
            n176 = Decimate 1D Array(w423) -> (w407:cluster{dbl[], dbl[]}[], w408:cluster{dbl[], dbl[]}[])
            n177 = local read "Slider Min"() -> (w404:dbl)
            n178 = local read "Sat-Trans Slider"() -> (w402:dbl)
            n179 = Array To Cluster(array=w407) -> (cluster=w422:T22)
            n180 = local read "New: Dielectric"() -> (w417:dbl)
            n181 = local read "Num Pts"() -> (w400:dbl)
            n182 = local read "New: Width"() -> (w419:dbl)
            n183 = local read "New: Length"() -> (w418:dbl)
            n184 = Unbundle(w422) -> ("[0]"=w421:cluster{dbl[], dbl[]})  [unwired: 8 out]
            n185 = Absolute Value(x=w404) -> (abs(x)=w403:dbl)
            n186 = Unbundle(w421) -> (w405:dbl[], w420:dbl[])
            n187 = Add(x=w402, y=w403) -> (x+y=w401:dbl)
            n188 = Array Subset(array=w405, index=w401, length=w400) -> (w415:dbl[])
            n189 = local write "Sat Vg Array-Used"(w415) -> ()
            n190 = Array Subset(array=w420, index=w401, length=w400) -> (w416:dbl[])
            n191 = call "Mobility-Vt-Used Pts_Saturation.vi"("Width"=w419, "Length"=w418, "Dielectric (d)"=w417, "Sat Id Used"=w416, "Vg Used"=w415) -> ("Vt"=w411:dbl, "Mobility"=w412:dbl)  [unwired: 4 in, 1 out]
            n192 = local write "Index-Sat"(w401) -> ()
            n193 = local write "Sat Id-Used"(w416) -> ()
            n194 = Bundle(w415, w416) -> (w409:cluster{dbl[], dbl[]})  [unwired: 1 in]
            n195 = local read "Re-Calculated Values Cluster"() -> (w414:T9)
            n196 = Bundle By Name(cluster=w414, "Mobility-Sat"=w412, "Vt-Sat"=w411) -> (w413:T9)
            n197 = local write "Re-Calculated Values Cluster"(w413) -> ()
            n198 = Build Array (concatenate)(w407, w408, w409) -> (w406:cluster{dbl[], dbl[]}[])
            n199 = local write "Sqrt-Sat"(w406) -> ()
          }
          event "Lin-Trans Slider": Value Change {
            n200 = event-data() -> ()  [unwired: 1 in, 5 out]
            n201 = local read "Sqrt-Lin"() -> (w447:cluster{dbl[], dbl[]}[])
            n202 = Decimate 1D Array(w447) -> (w432:cluster{dbl[], dbl[]}[], w433:cluster{dbl[], dbl[]}[])
            n203 = local read "Slider Min"() -> (w429:dbl)
            n204 = Array To Cluster(array=w432) -> (cluster=w446:T22)
            n205 = local read "Lin-Trans Slider"() -> (w427:dbl)
            n206 = local read "New: Dielectric"() -> (w440:dbl)
            n207 = local read "Num Pts"() -> (w443:dbl)
            n208 = local read "New: Width"() -> (w442:dbl)
            n209 = local read "New: Length"() -> (w441:dbl)
            n210 = local read "Lin Vd"() -> (w424:dbl)
            n211 = Unbundle(w446) -> ("[0]"=w445:cluster{dbl[], dbl[]})  [unwired: 8 out]
            n212 = Absolute Value(x=w429) -> (abs(x)=w428:dbl)
            n213 = Unbundle(w445) -> (w430:dbl[], w444:dbl[])
            n214 = Add(x=w427, y=w428) -> (x+y=w426:dbl)
            n215 = Array Subset(array=w430, index=w426, length=w443) -> (w438:dbl[])
            n216 = local write "Lin-Vg Array-Used"(w438) -> ()
            n217 = Array Subset(array=w444, index=w426, length=w443) -> (w439:dbl[])
            n218 = call "Mobility-Vt-Used Pts_Linear.vi"("Width"=w442, "Length"=w441, "Vd"=w424, "Dielectric (d)"=w440, "Id Used"=w439, "Vg Used"=w438) -> ("Mobility"=w435:dbl)  [unwired: 3 in, 2 out]
            n219 = local write "Index-Lin"(w426) -> ()
            n220 = local write "Lin Id-Used"(w439) -> ()
            n221 = Bundle(w438, w439) -> (w434:cluster{dbl[], dbl[]})  [unwired: 1 in]
            n222 = local read "Re-Calculated Values Cluster"() -> (w437:T9)
            n223 = Bundle By Name(cluster=w437, "Moblitity-Lin"=w435) -> (w436:T9)
            n224 = local write "Re-Calculated Values Cluster"(w436) -> ()
            n225 = Build Array (concatenate)(w432, w433, w434) -> (w431:cluster{dbl[], dbl[]}[])
            n226 = local write "Sqrt-Lin"(w431) -> ()
          }
          event "Sat-Log Slider": Value Change {
            n227 = event-data() -> ()  [unwired: 1 in, 5 out]
            n228 = local read "Log-Sat"() -> (w449:cluster{dbl[], dbl[]}[])
            n229 = Decimate 1D Array(w449) -> (w457:cluster{dbl[], dbl[]}[], w458:cluster{dbl[], dbl[]}[])
            n230 = local read "Slider Min"() -> (w455:dbl)
            n231 = Array To Cluster(array=w457) -> (cluster=w467:T22)
            n232 = local read "Num Pts Log"() -> (w464:dbl)
            n233 = local read "Sat-Log Slider"() -> (w453:dbl)
            n234 = Unbundle(w467) -> ("[0]"=w466:cluster{dbl[], dbl[]})  [unwired: 8 out]
            n235 = Absolute Value(x=w455) -> (abs(x)=w454:dbl)
            n236 = Unbundle(w466) -> (w456:dbl[], w465:dbl[])
            n237 = Add(x=w453, y=w454) -> (x+y=w451:dbl)
            n238 = Array Subset(array=w456, index=w451, length=w464) -> (w462:dbl[])
            n239 = Array Subset(array=w465, index=w451, length=w464) -> (w463:dbl[])
            n240 = local write "Vg Array-Log-Used"(w462) -> ()
            n241 = local write "IndexLog-Sat"(w451) -> ()
            n242 = Bundle(w462, w463) -> (w450:cluster{dbl[], dbl[]})  [unwired: 1 in]
            n243 = call "STS-Used.vi"("Id Used"=w463, "Vg-Used"=w462) -> ("STS"=w459:dbl)  [unwired: 9 in]
            n244 = local write "Sat Id-Log-Used"(w463) -> ()
            n245 = local read "Re-Calculated Values Cluster"() -> (w461:T9)
            n246 = Bundle By Name(cluster=w461, "STS"=w459) -> (w460:T9)
            n247 = local write "Re-Calculated Values Cluster"(w460) -> ()
            n248 = Build Array (concatenate)(w457, w458, w450) -> (w448:cluster{dbl[], dbl[]}[])
            n249 = local write "Log-Sat"(w448) -> ()
          }
          event "Lin-Log Slider": Value Change {
            # "No Indicator for Lin-Log Slider Use"
            n250 = event-data() -> ()  [unwired: 1 in, 5 out]
            n251 = local read "Log-Lin"() -> (w471:cluster{dbl[], dbl[]}[])
            n252 = Decimate 1D Array(w471) -> (w477:cluster{dbl[], dbl[]}[], w478:cluster{dbl[], dbl[]}[])
            n253 = local read "Slider Min"() -> (w474:dbl)
            n254 = Array To Cluster(array=w477) -> (cluster=w484:T22)
            n255 = local read "Num Pts Log"() -> (w481:dbl)
            n256 = local read "Lin-Log Slider"() -> (w472:dbl)
            n257 = Unbundle(w484) -> ("[0]"=w483:cluster{dbl[], dbl[]})  [unwired: 8 out]
            n258 = Absolute Value(x=w474) -> (abs(x)=w473:dbl)
            n259 = Unbundle(w483) -> (w475:dbl[], w482:dbl[])
            n260 = Add(x=w472, y=w473) -> (x+y=w470:dbl)
            n261 = Array Subset(array=w475, index=w470, length=w481) -> (w479:dbl[])
            n262 = local write "Lin-Vg Array-Log Used"(w479) -> ()
            n263 = Array Subset(array=w482, index=w470, length=w481) -> (w480:dbl[])
            n264 = local write "IndexLog-Sat"(w470) -> ()
            n265 = Bundle(w479, w480) -> (w469:cluster{dbl[], dbl[]})  [unwired: 1 in]
            n266 = call "STS-Used.vi"("Id Used"=w480, "Vg-Used"=w479) -> ()  [unwired: 9 in, 1 out]
            n267 = local write "Lin Id-Log Used"(w480) -> ()
            n268 = Build Array (concatenate)(w477, w478, w469) -> (w476:cluster{dbl[], dbl[]}[])
            n269 = local write "Log-Lin"(w476) -> ()
          }
          event "Include Images?": Value Change {
            n270 = event-data() -> ()  [unwired: 1 in, 5 out]
          }
        }
      }
      frame "Read Data" {
        n271 = call "Recorded Values.vi"("Path"=w529) -> ("Recorded Char"=w547:T9, "Recorded Prop"=w537:T1, "Fabrication Prop"=w531:T4)  [unwired: 8 in]
        n272 = Strip Path(path=w529) -> (stripped path=w530:path, name=w528:string)
        n273 = local write "Fabrication Prop"(w531) -> ()
        n274 = local write "Recorded Prop"(w537) -> ()
        n275 = Unbundle By Name(w537) -> ("Date Recorded"=w536:string, "Index"=w534:string, "Length"=w535:dbl, "Width"=w533:dbl, "Sample Temp"=w532:dbl)
        n276 = local write "Recorded Values Cluster"(w547) -> ()
        n277 = Unbundle By Name(w537) -> ("Sample Temp"=w540:dbl)
        n278 = Unbundle By Name(w531) -> ("Dielectric (nm)"=w525:dbl, "Comments"=w524:string)
        n279 = List Folder(path=w530) -> (filenames=w526:string[])  [unwired: 3 in, 3 out]
        n280 = local write "Rec: Dielectric (d)"(w525) -> ()
        n281 = local write "Date Created"(w536) -> ()
        n282 = local write "Index"(w534) -> ()
        n283 = local write "Rec: Length"(w535) -> ()
        n284 = local write "Rec: Width"(w533) -> ()
        n285 = local write "Rec: Temp"(w532) -> ()
        n286 = Equal To 0?(x=w540) -> (x = 0?=w543:bool)
        n287 = Number To Decimal String(number=w540) -> (decimal integer string=w544:string)  [unwired: 1 in]
        n288 = local write "Comments:"(w524) -> ()
        n289 = Search 1D Array(1D array=w526, element=w528) -> (index of element=w523:i32)  [unwired: 1 in]
        n290 = Equal?(x="", y=w544) -> (x = y?=w542:bool)
        n291 = Index Array(array=w526, index=w523) -> (element=w527:string)
        n292 = Or(x=w543, y=w542) -> (x .or. y?=w541:bool)
        n293 = local write "Data Name:"(w527) -> ()
        n294 = case shown="False" w541 {
          tunnel: [w548 w549] -> w538
          tunnel: w540 -> [w548 _]
          frame False {
          }
          frame True {
            n295 = local read "Room Temp"() -> (w549:dbl)
          }
        }
        n296 = local write "New: Temp"(w538) -> ()
        n297 = Bundle By Name(cluster=w537, "Sample Temp"=w538) -> (w539:T1)
        n298 = local write "Recorded Prop"(w539) -> ()
      }
      frame "Calculated Values" {
        n299 = case shown="True" "Include Transport?" {
          tunnel: w561 -> [_ w611]
          frame False {
          }
          frame True {
            n300 = local read "Transport Style Controls"() -> (w610:T10)
            n301 = call "TRF to TSP Plot.vi"("Transport Graph Properties"=w610, "Transfer File"=w611) -> ("Transport"=w609:cluster{ext[], ext[]}[])  [unwired: 7 in, 2 out]
            n302 = Array Size(array=w609) -> (size(s)=w608:i32)
            n303 = local write "Transport"(w609) -> ()
            n304 = for {
              N: w608 -> [_]
              tunnel: w610 -> [w615]
              i -> [w614]
              n305 = Unbundle By Name(w615) -> ("Transport Line Size"=w612:u16, "Transport Line Color"=w613:u32)
              n306 = property on="Transport" class="XYGraph (strict)"("Active Plot"=w614, "Plot.Plot Color"=w613, "Plot.Line Width"=w612) -> ()  [unwired: 2 in, 2 out]
            }
          }
        }
        n307 = local read "Fabrication Prop"() -> (w590:T4)
        n308 = local read "Recorded Prop"() -> (w583:T1)
        n309 = call "Mobility-Vt Calculator-File.vi"("NumPts"=w585, "Path"=w561) -> ("Used Points"=w578:T23, "Graph Cluster"=w567:T24, "Lin Vd"=w574:dbl, "Output"=w598:T25)  [unwired: 6 in]
        n310 = call "STS Calculator-File.vi"("NumPts"=w584, "Path"=w561) -> ("Used Points"=w572:T26, "XY Graph-Sat"=w551:cluster{dbl[], dbl[]}[], "XY Graph-Lin"=w555:cluster{dbl[], dbl[]}[], "Ouput"=w593:cluster{"STS-Sat":dbl, "STS-Lin":dbl})  [unwired: 6 in]
        n311 = Unbundle By Name(w590) -> ("Dielectric (nm)"=w588:dbl)
        n312 = Unbundle By Name(w583) -> ("Sample Temp"=w582:dbl)
        n313 = Unbundle By Name(w598) -> ("Mobility-Sat"=w597:dbl, "Vt-Sat"=w589:dbl, "Mobility-Lin"=w596:dbl, "Off I-Sat"=w595:dbl, "On/Off I-Sat"=w594:dbl)  [unwired: 1 out]
        n314 = local write "Lin Vd"(w574) -> ()
        n315 = local write "Log-Sat"(w551) -> ()
        n316 = Unbundle By Name(w593) -> ("STS-Sat"=w587:dbl)  [unwired: 1 out]
        n317 = local write "Log-Lin"(w555) -> ()
        n318 = case shown="True" w550 {
          tunnel: w581 -> [_ w607]
          tunnel: w580 -> [_ w606]
          tunnel: w561 -> [_ w605]
          frame False {
          }
          frame True {
            n319 = call "Image from TRF Display.vi"("No Image File"=w606, "Image Folder"=w607, "Transfer File"=w605) -> ("Image Out 2"=w601:T8, "Image Out"=w602:T8, "Image File"=w603:path, "Image Name"=w604:string)  [unwired: 5 in]
            n320 = local write "Image File"(w603) -> ()
            n321 = local write "Image Name"(w604) -> ()
            n322 = local write "Image Out"(w602) -> ()
            n323 = local write "Image Preview"(w601) -> ()
          }
        }
        n324 = call "Trap Density_VT.vi"("VT"=w589, "Dielectric"=w588) -> ("Trap Density-VT"=w592:dbl)
        n325 = call "Trap Density_STS.vi"("Temp (T) [K]"=w582, "S.T.S. (S)"=w587, "Dielectric"=w588) -> ("Trap Density (N)"=w591:dbl)  [unwired: 8 in]
        n326 = local read "Calculated Values Cluster"() -> (w600:T9)
        n327 = Bundle By Name(cluster=w600, "Mobility-Sat"=w597, "Moblitity-Lin"=w596, "On/Off"=w594, "Off Current"=w595, "Vt-Sat"=w589, "STS"=w587, "Trap Density-VT"=w592, "Trap Density-STS"=w591) -> (w599:T9)
        n328 = Unbundle By Name(w572) -> ("Sat Vg Used"=w571:dbl[], "Sat Log(Id) Used"=w570:dbl[], "Lin Vg Used"=w569:dbl[], "Lin Log(Id) Used"=w568:dbl[], "STS Index-Sat"=w553:dbl, "STS Index-Lin"=w554:dbl)
        n329 = Unbundle By Name(w578) -> ("Sat Vg Used"=w577:dbl[], "Sat Sqrt(Id) Used"=w576:dbl[], "Lin Vg Used"=w575:dbl[], "Lin Sqrt(Id) Used"=w573:dbl[], "Index-Lin"=w563:dbl, "Index-Sat"=w562:dbl)
        n330 = local write "Vg Array-Log-Used"(w571) -> ()
        n331 = local write "Sat Id-Log-Used"(w570) -> ()
        n332 = local write "Lin-Vg Array-Log Used"(w569) -> ()
        n333 = local write "Lin Id-Log Used"(w568) -> ()
        n334 = local write "IndexLog-Sat"(w553) -> ()
        n335 = local write "Index-Lin"(w554) -> ()
        n336 = local write "Calculated Values Cluster"(w599) -> ()
        n337 = local write "Sat Vg Array-Used"(w577) -> ()
        n338 = local write "Sat Id-Used"(w576) -> ()
        n339 = local write "Lin-Vg Array-Used"(w575) -> ()
        n340 = local write "Lin Id-Used"(w573) -> ()
        n341 = local write "Index-Sat"(w562) -> ()
        n342 = local write "Index-Lin"(w563) -> ()
        n343 = local write "Lin-Log Slider"(w554) -> ()
        n344 = local write "Sat-Log Slider"(w553) -> ()
        n345 = local write "Sat-Trans Slider"(w562) -> ()
        n346 = local write "Lin-Trans Slider"(w563) -> ()
        n347 = Unbundle By Name(w567) -> ("Raw Sat"=w560:cluster{dbl[], dbl[]}[], "Sqrt Sat"=w564:cluster{dbl[], dbl[]}[], "Raw Lin"=w566:cluster{dbl[], dbl[]}[], "Sqrt Lin"=w565:cluster{dbl[], dbl[]}[])
        n348 = Index Array(array=w560) -> (element=w559:cluster{dbl[], dbl[]})  [unwired: 1 in]
        n349 = Unbundle(w559) -> (w558:dbl[])  [unwired: 1 out]
        n350 = Array Max & Min(array=w558) -> (max value=w557:dbl, min value=w556:dbl)  [unwired: 2 out]
        n351 = property on="Sat-Trans Slider" class="Slide (strict)"("Scale.Maximum"=w557, "Scale.Minimum"=w556) -> ()  [unwired: 2 in, 2 out]
        n352 = property on="Lin-Trans Slider" class="Slide (strict)"("Scale.Maximum"=w557, "Scale.Minimum"=w556) -> ()  [unwired: 2 in, 2 out]
        n353 = property on="Sat-Log Slider" class="Slide (strict)"("Scale.Maximum"=w557, "Scale.Minimum"=w556) -> ()  [unwired: 2 in, 2 out]
        n354 = property on="Lin-Log Slider" class="Slide (strict)"("Scale.Maximum"=w557, "Scale.Minimum"=w556) -> ()  [unwired: 2 in, 2 out]
        n355 = local write "Slider Max"(w557) -> ()
        n356 = local write "Slider Min"(w556) -> ()
        n357 = local write "Raw- Sat"(w560) -> ()
        n358 = local write "Raw- Lin"(w566) -> ()
        n359 = local write "Sqrt-Sat"(w564) -> ()
        n360 = local write "Sqrt-Lin"(w565) -> ()
      }
      frame "Re-Calculated Values" {
        n361 = local read "Vg Array-Log-Used"() -> (w624:dbl[])
        n362 = local read "Sat Vg Array-Used"() -> (w632:dbl[])
        n363 = local read "Lin-Vg Array-Used"() -> (w638:dbl[])
        n364 = local read "Sat Id-Log-Used"() -> (w623:dbl[])
        n365 = local read "New: Dielectric"() -> (w636:dbl)
        n366 = local read "New: Dielectric"() -> (w621:dbl)
        n367 = local read "New: Length"() -> (w635:dbl)
        n368 = local read "New: Length"() -> (w631:dbl)
        n369 = local read "New: Width"() -> (w634:dbl)
        n370 = local read "New: Width"() -> (w630:dbl)
        n371 = local read "Lin Id-Used"() -> (w637:dbl[])
        n372 = local read "Sat Id-Used"() -> (w629:dbl[])
        n373 = local read "Re-Calculated Values Cluster"() -> (w640:T9)
        n374 = local read "New: Dielectric"() -> (w620:dbl)
        n375 = local read "New: Temp"() -> (w619:dbl)
        n376 = local read "Lin Vd"() -> (w616:dbl)
        n377 = call "Mobility-Vt-Used Pts_Saturation.vi"("Width"=w630, "Length"=w631, "Dielectric (d)"=w621, "Sat Id Used"=w629, "Vg Used"=w632) -> ("Vt"=w627:dbl, "Mobility"=w628:dbl)  [unwired: 4 in, 1 out]
        n378 = call "STS-Used.vi"("Id Used"=w623, "Vg-Used"=w624) -> ("STS"=w622:dbl)  [unwired: 9 in]
        n379 = call "Mobility-Vt-Used Pts_Linear.vi"("Width"=w634, "Length"=w635, "Vd"=w616, "Dielectric (d)"=w636, "Id Used"=w637, "Vg Used"=w638) -> ("Mobility"=w633:dbl)  [unwired: 3 in, 2 out]
        n380 = call "Trap Density_VT.vi"("VT"=w627, "Dielectric"=w621) -> ("Trap Density-VT"=w626:dbl)
        n381 = call "Trap Density_STS.vi"("Temp (T) [K]"=w619, "S.T.S. (S)"=w622, "Dielectric"=w620) -> ("Trap Density (N)"=w618:dbl)  [unwired: 8 in]
        n382 = Bundle By Name(cluster=w640, "Mobility-Sat"=w628, "Moblitity-Lin"=w633, "Vt-Sat"=w627, "STS"=w622, "Trap Density-VT"=w626, "Trap Density-STS"=w618) -> (w639:T9)
        n383 = local write "Re-Calculated Values Cluster"(w639) -> ()
      }
      frame "Next File" {
        n384 = Strip Path(path=w657) -> (stripped path=w647:path, name=w655:string)
        n385 = local write "Transfer Folder"(w647) -> ()
        n386 = List Folder(path=w647) -> (filenames=w641:string[], error out=w650:errorcluster)  [unwired: 3 in, 2 out]
        n387 = Array Size(array=w641) -> (size(s)=w654:i32)
        n388 = Search 1D Array(1D array=w641, element=w655) -> (index of element=w652:i32)  [unwired: 1 in]
        n389 = Decrement(x=w654) -> (x-1=w653:i32)
        n390 = Equal?(x=w653, y=w652) -> (x = y?=w651:bool)
        n391 = case shown="False" w651 {
          tunnel: w643 -> [w660 _]
          tunnel: [w659 0] -> w642
          tunnel: w650 -> [w658 w661]
          tunnel: [w658 w661] -> _
          frame False {
            n392 = Increment(x=w660) -> (x+1=w659:i32)
          }
          frame True {
          }
        }
        n393 = Path To String(path=w647) -> (string=w648:string)
        n394 = Index Array(array=w641, index=w642) -> (element=w649:string)
        n395 = Concatenate Strings(w648, "\\", w649) -> (w645:string)
        n396 = String To Path(string=w645) -> (path=w644:path)
        n397 = local write "Transfer File"(w644) -> ()
      }
      frame "Previous File" {
        n398 = Strip Path(path=w669) -> (stripped path=w666:path, name=w678:string)
        n399 = local write "Transfer Folder"(w666) -> ()
        n400 = List Folder(path=w666) -> (filenames=w670:string[], error out=w675:errorcluster)  [unwired: 3 in, 2 out]
        n401 = Array Size(array=w670) -> (size(s)=w664:i32)
        n402 = Search 1D Array(1D array=w670, element=w678) -> (index of element=w677:i32)  [unwired: 1 in]
        n403 = Decrement(x=w664) -> (x-1=w663:i32)
        n404 = Equal To 0?(x=w677) -> (x = 0?=w676:bool)
        n405 = case shown="False" w676 {
          tunnel: w668 -> [w682 _]
          tunnel: [w681 w683] -> w667
          tunnel: w675 -> [w680 w684]
          tunnel: [w680 w684] -> _
          tunnel: w663 -> [_ w683]
          frame False {
            n406 = Decrement(x=w682) -> (x-1=w681:i32)
          }
          frame True {
          }
        }
        n407 = Path To String(path=w666) -> (string=w665:string)
        n408 = Index Array(array=w670, index=w667) -> (element=w674:string)
        n409 = Concatenate Strings(w665, "\\", w674) -> (w672:string)
        n410 = String To Path(string=w672) -> (path=w671:path)
        n411 = local write "Transfer File"(w671) -> ()
      }
      frame "Discard File" {
      }
      frame "Save" {
        n412 = stacked-sequence {
          seq-local: [w702 _] -> [_ w1199]
          seq-local: [w701 _] -> [_ w1197]
          tunnel: w693 -> [w703 w1200]
          frame #0 {
            # "Saves each Re-calculated parameter in sequence"
            n413 = stacked-sequence {
              tunnel: [_ _ _ _ _ _ _ _ _ _ _ _ _ w1167] -> w701
              tunnel: w703 -> [w723 _ _ _ _ _ _ _ _ _ _ _ _ _]
              frame #0 {
                n414 = call-poly <vilib>:"Read From Spreadsheet File.vi"("file path (dialog if empty)"=w723) -> ("all rows"=w722:string[][])  [unwired: 6 in, 4 out]
                n415 = Array Size(array=w722) -> (size(s)=w727:i32[])
                n416 = Array Subset(array=w722, index (row)=0, index (col)=0, length (col)=3) -> (w731:string[][])  [unwired: 1 in]
                n417 = Index Array(array=w727, index=0) -> (element=w725:i32)
                n418 = Reshape Array(w731, w725) -> (w724:string[])
                n419 = Search 1D Array(1D array=w724, element="Dielectric (nm):") -> (index of element=w734:i32)  [unwired: 1 in]
                n420 = Equal?(x=w734, y=-1) -> (x = y?=w733:bool)
                n421 = case shown="False" w733 {
                  tunnel: w722 -> [w742 w746]
                  tunnel: w734 -> [w738 _]
                  tunnel: [w737 w746] -> w732
                  frame False {
                    n422 = local read "Rec: Dielectric (d)"() -> (w744:dbl)
                    n423 = Number To Fractional String(number=w744) -> (F-format string=w739:string)  [unwired: 3 in]
                    n424 = Divide(x=w738, y=3) -> (x/y=w741:dbl)
                    n425 = To Word Integer(number=w741) -> (16bit integer=w740:i16)
                    n426 = Replace Array Subset(array=w742, new element=w739, index (row)=w740, index (col)=1) -> (w737:string[][])
                  }
                  frame True {
                  }
                }
                n427 = local write "Save Array"(w732) -> ()
              }
              frame #1 {
                n428 = local read "Save Array"() -> (w748:string[][])
                n429 = Array Size(array=w748) -> (size(s)=w751:i32[])
                n430 = Array Subset(array=w748, index (row)=0, index (col)=0, length (col)=3) -> (w755:string[][])  [unwired: 1 in]
                n431 = Index Array(array=w751, index=0) -> (element=w749:i32)
                n432 = Reshape Array(w755, w749) -> (w747:string[])
                n433 = Search 1D Array(1D array=w747, element="Comments:") -> (index of element=w758:i32)  [unwired: 1 in]
                n434 = Equal?(x=w758, y=-1) -> (x = y?=w757:bool)
                n435 = case shown="False" w757 {
                  tunnel: w748 -> [w766 w769]
                  tunnel: w758 -> [w763 _]
                  tunnel: [w762 w769] -> w756
                  frame False {
                    n436 = local read "New: Comments"() -> (w761:string)
                    n437 = Divide(x=w763, y=3) -> (x/y=w765:dbl)
                    n438 = To Word Integer(number=w765) -> (16bit integer=w764:i16)
                    n439 = Replace Array Subset(array=w766, new element=w761, index (row)=w764, index (col)=1) -> (w762:string[][])
                  }
                  frame True {
                  }
                }
                n440 = local write "Save Array"(w756) -> ()
              }
              frame #2 {
                n441 = local read "Save Array"() -> (w771:string[][])
                n442 = Array Size(array=w771) -> (size(s)=w774:i32[])
                n443 = Array Subset(array=w771, index (row)=0, index (col)=0, length (col)=3) -> (w778:string[][])  [unwired: 1 in]
                n444 = Index Array(array=w774, index=0) -> (element=w772:i32)
                n445 = Reshape Array(w778, w772) -> (w770:string[])
                n446 = Search 1D Array(1D array=w770, element="Length (um):") -> (index of element=w781:i32)  [unwired: 1 in]
                n447 = Equal?(x=w781, y=-1) -> (x = y?=w780:bool)
                n448 = case shown="False" w780 {
                  tunnel: w771 -> [w791 w794]
                  tunnel: w781 -> [w788 _]
                  tunnel: [w787 w794] -> w779
                  frame False {
                    n449 = local read "New: Length"() -> (w784:dbl)
                    n450 = Divide(x=w788, y=3) -> (x/y=w790:dbl)
                    n451 = Format Value(format string="%#g", value (0)=w784) -> (output string=w785:string)  [unwired: 1 in]
                    n452 = To Word Integer(number=w790) -> (16bit integer=w789:i16)
                    n453 = Replace Array Subset(array=w791, new element=w785, index (row)=w789, index (col)=1) -> (w787:string[][])
                  }
                  frame True {
                  }
                }
                n454 = local write "Save Array"(w779) -> ()
              }
              frame #3 {
                n455 = local read "Save Array"() -> (w796:string[][])
                n456 = Array Size(array=w796) -> (size(s)=w801:i32[])
                n457 = Array Subset(array=w796, index (row)=0, index (col)=0, length (col)=3) -> (w797:string[][])  [unwired: 1 in]
                n458 = Index Array(array=w801, index=0) -> (element=w803:i32)
                n459 = Reshape Array(w797, w803) -> (w795:string[])
                n460 = Search 1D Array(1D array=w795, element="Width (um):") -> (index of element=w806:i32)  [unwired: 1 in]
                n461 = Equal?(x=w806, y=-1) -> (x = y?=w805:bool)
                n462 = case shown="False" w805 {
                  tunnel: w806 -> [w814 _]
                  tunnel: w796 -> [w813 w819]
                  tunnel: [w812 w819] -> w804
                  frame False {
                    n463 = local read "New: Width"() -> (w809:dbl)
                    n464 = Divide(x=w814, y=3) -> (x/y=w816:dbl)
                    n465 = To Word Integer(number=w816) -> (16bit integer=w815:i16)
                    n466 = Format Value(format string="%#g", value (0)=w809) -> (output string=w810:string)  [unwired: 1 in]
                    n467 = Replace Array Subset(array=w813, new element=w810, index (row)=w815, index (col)=1) -> (w812:string[][])
                  }
                  frame True {
                  }
                }
                n468 = local write "Save Array"(w804) -> ()
              }
              frame #4 {
                w829 = "Sample Temp (K):"
                n469 = local read "Save Array"() -> (w821:string[][])
                n470 = Array Size(array=w821) -> (size(s)=w826:i32[])
                n471 = Array Subset(array=w821, index (row)=0, index (col)=0, length (col)=3) -> (w822:string[][])  [unwired: 1 in]
                n472 = Index Array(array=w826, index=0) -> (element=w828:i32)
                n473 = Reshape Array(w822, w828) -> (w820:string[])
                n474 = Search 1D Array(1D array=w820, element=w829) -> (index of element=w832:i32)  [unwired: 1 in]
                n475 = Equal?(x=w832, y=-1) -> (x = y?=w831:bool)
                n476 = case shown="False" w831 {
                  tunnel: w821 -> [w841 w855]
                  tunnel: w832 -> [w838 _]
                  tunnel: [w837 w854] -> w830
                  tunnel: w820 -> [_ w857]
                  tunnel: w829 -> [_ w844]
                  frame False {
                    n477 = local read "New: Temp"() -> (w835:dbl)
                    n478 = Divide(x=w838, y=3) -> (x/y=w840:dbl)
                    n479 = Format Value(format string="%#g", value (0)=w835) -> (output string=w834:string)  [unwired: 1 in]
                    n480 = To Word Integer(number=w840) -> (16bit integer=w839:i16)
                    n481 = Replace Array Subset(array=w841, new element=w834, index (row)=w839, index (col)=1) -> (w837:string[][])
                  }
                  frame True {
                    n482 = local read "New: Temp"() -> (w846:dbl)
                    n483 = Search 1D Array(1D array=w857, element="Width (um):") -> (index of element=w851:i32)  [unwired: 1 in]
                    n484 = Divide(x=w851, y=3) -> (x/y=w852:dbl)
                    n485 = To Word Integer(number=w852) -> (16bit integer=w850:i16)
                    n486 = Format Value(format string="%#g", value (0)=w846) -> (output string=w845:string)  [unwired: 1 in]
                    n487 = Build Array(w844, w845) -> (w848:string[])
                    n488 = Increment(x=w850) -> (x+1=w849:i16)
                    n489 = Insert Into Array(array=w855, index (row)=w849, new element=w848) -> (w854:string[][])  [unwired: 1 in]
                  }
                }
                n490 = local write "Save Array"(w830) -> ()
              }
              frame #5 {
                w867 = "Mobility-Sat (cm^2/Vs):"
                n491 = local read "Save Array"() -> (w859:string[][])
                n492 = Array Size(array=w859) -> (size(s)=w864:i32[])
                n493 = Array Subset(array=w859, index (row)=0, index (col)=0, length (col)=3) -> (w860:string[][])  [unwired: 1 in]
                n494 = Index Array(array=w864, index=0) -> (element=w866:i32)
                n495 = Reshape Array(w860, w866) -> (w858:string[])
                n496 = Search 1D Array(1D array=w858, element=w867) -> (index of element=w870:i32)  [unwired: 1 in]
                n497 = Equal?(x=w870, y=-1) -> (x = y?=w869:bool)
                n498 = case shown="False" w869 {
                  tunnel: w859 -> [w880 w890]
                  tunnel: w870 -> [w877 _]
                  tunnel: [w876 w889] -> w868
                  tunnel: w858 -> [_ w887]
                  tunnel: w867 -> [_ w885]
                  frame False {
                    n499 = local read "Re-Calculated Values Cluster"() -> (w873:T9)
                    n500 = Unbundle By Name(w873) -> ("Mobility-Sat"=w872:dbl)
                    n501 = Divide(x=w877, y=3) -> (x/y=w879:dbl)
                    n502 = To Word Integer(number=w879) -> (16bit integer=w878:i16)
                    n503 = Format Value(format string="%#g", value (0)=w872) -> (output string=w874:string)  [unwired: 1 in]
                    n504 = Replace Array Subset(array=w880, new element=w874, index (row)=w878, index (col)=1) -> (w876:string[][])
                  }
                  frame True {
                    n505 = local read "Re-Calculated Values Cluster"() -> (w884:T9)
                    n506 = Unbundle By Name(w884) -> ("Mobility-Sat"=w883:dbl)
                    n507 = Search 1D Array(1D array=w887, element="Mobility (cm^2/Vs):") -> (index of element=w893:i32)  [unwired: 1 in]
                    n508 = Divide(x=w893, y=3) -> (x/y=w894:dbl)
                    n509 = To Word Integer(number=w894) -> (16bit integer=w886:i16)
                    n510 = Format Value(format string="%#g", value (0)=w883) -> (output string=w888:string)  [unwired: 1 in]
                    n511 = Build Array(w885, w888) -> (w892:string[])
                    n512 = Replace Array Subset(array=w890, new element=w892, index (row)=w886) -> (w889:string[][])  [unwired: 1 in]
                  }
                }
                n513 = local write "Save Array"(w868) -> ()
              }
              frame #6 {
                w906 = "Mobility-Lin (cm^2/Vs):"
                n514 = local read "Save Array"() -> (w897:string[][])
                n515 = Array Size(array=w897) -> (size(s)=w903:i32[])
                n516 = Array Subset(array=w897, index (row)=0, index (col)=0, length (col)=3) -> (w899:string[][])  [unwired: 1 in]
                n517 = Index Array(array=w903, index=0) -> (element=w905:i32)
                n518 = Reshape Array(w899, w905) -> (w898:string[])
                n519 = Search 1D Array(1D array=w898, element=w906) -> (index of element=w909:i32)  [unwired: 1 in]
                n520 = Equal?(x=w909, y=-1) -> (x = y?=w908:bool)
                n521 = case shown="True" w908 {
                  tunnel: w897 -> [w919 w927]
                  tunnel: w909 -> [w916 _]
                  tunnel: [w915 w926] -> w907
                  tunnel: w898 -> [_ w925]
                  tunnel: w906 -> [_ w924]
                  frame False {
                    n522 = local read "Re-Calculated Values Cluster"() -> (w912:T9)
                    n523 = Unbundle By Name(w912) -> ("Moblitity-Lin"=w911:dbl)
                    n524 = Divide(x=w916, y=3) -> (x/y=w918:dbl)
                    n525 = To Word Integer(number=w918) -> (16bit integer=w917:i16)
                    n526 = Format Value(format string="%#g", value (0)=w911) -> (output string=w913:string)  [unwired: 1 in]
                    n527 = Replace Array Subset(array=w919, new element=w913, index (row)=w917, index (col)=1) -> (w915:string[][])
                  }
                  frame True {
                    n528 = local read "Re-Calculated Values Cluster"() -> (w923:T9)
                    n529 = Unbundle By Name(w923) -> ("Moblitity-Lin"=w922:dbl)
                    n530 = Search 1D Array(1D array=w925, element="Mobility-Sat (cm^2/Vs):") -> (index of element=w932:i32)  [unwired: 1 in]
                    n531 = Divide(x=w932, y=3) -> (x/y=w933:dbl)
                    n532 = To Word Integer(number=w933) -> (16bit integer=w931:i16)
                    n533 = Format Value(format string="%#g", value (0)=w922) -> (output string=w936:string)  [unwired: 1 in]
                    n534 = Build Array(w924, w936) -> (w929:string[])
                    n535 = Increment(x=w931) -> (x+1=w930:i16)
                    n536 = Insert Into Array(array=w927, index (row)=w930, new element=w929) -> (w926:string[][])  [unwired: 1 in]
                  }
                }
                n537 = local write "Save Array"(w907) -> ()
              }
              frame #7 {
                w946 = "On/Off I-Sat:"
                n538 = local read "Save Array"() -> (w937:string[][])
                n539 = Array Size(array=w937) -> (size(s)=w943:i32[])
                n540 = Array Subset(array=w937, index (row)=0, index (col)=0, length (col)=3) -> (w939:string[][])  [unwired: 1 in]
                n541 = Index Array(array=w943, index=0) -> (element=w945:i32)
                n542 = Reshape Array(w939, w945) -> (w938:string[])
                n543 = Search 1D Array(1D array=w938, element=w946) -> (index of element=w949:i32)  [unwired: 1 in]
                n544 = Equal?(x=w949, y=-1) -> (x = y?=w948:bool)
                n545 = case shown="True" w948 {
                  tunnel: w937 -> [w959 w968]
                  tunnel: w949 -> [w956 _]
                  tunnel: [w955 w969] -> w947
                  tunnel: w938 -> [_ w966]
                  tunnel: w946 -> [_ w964]
                  frame False {
                    n546 = local read "Re-Calculated Values Cluster"() -> (w952:T9)
                    n547 = Divide(x=w956, y=3) -> (x/y=w958:dbl)
                    n548 = Unbundle By Name(w952) -> ("On/Off"=w951:dbl)
                    n549 = To Word Integer(number=w958) -> (16bit integer=w957:i16)
                    n550 = Format Value(format string="%#g", value (0)=w951) -> (output string=w953:string)  [unwired: 1 in]
                    n551 = Replace Array Subset(array=w959, new element=w953, index (row)=w957, index (col)=1) -> (w955:string[][])
                  }
                  frame True {
                    n552 = local read "Re-Calculated Values Cluster"() -> (w963:T9)
                    n553 = Unbundle By Name(w963) -> ("On/Off"=w962:dbl)
                    n554 = Search 1D Array(1D array=w966, element="On/Off Current:") -> (index of element=w972:i32)  [unwired: 1 in]
                    n555 = Divide(x=w972, y=3) -> (x/y=w973:dbl)
                    n556 = To Word Integer(number=w973) -> (16bit integer=w965:i16)
                    n557 = Format Value(format string="%#g", value (0)=w962) -> (output string=w967:string)  [unwired: 1 in]
                    n558 = Build Array(w964, w967) -> (w971:string[])
                    n559 = Replace Array Subset(array=w968, new element=w971, index (row)=w965) -> (w969:string[][])  [unwired: 1 in]
                  }
                }
                n560 = local write "Save Array"(w947) -> ()
              }
              frame #8 {
                w985 = "Off I-Sat (A):"
                n561 = local read "Save Array"() -> (w976:string[][])
                n562 = Array Size(array=w976) -> (size(s)=w982:i32[])
                n563 = Array Subset(array=w976, index (row)=0, index (col)=0, length (col)=3) -> (w978:string[][])  [unwired: 1 in]
                n564 = Index Array(array=w982, index=0) -> (element=w984:i32)
                n565 = Reshape Array(w978, w984) -> (w977:string[])
                n566 = Search 1D Array(1D array=w977, element=w985) -> (index of element=w988:i32)  [unwired: 1 in]
                n567 = Equal?(x=w988, y=-1) -> (x = y?=w987:bool)
                n568 = case shown="True" w987 {
                  tunnel: w976 -> [w998 w1006]
                  tunnel: w988 -> [w995 _]
                  tunnel: [w994 w1005] -> w986
                  tunnel: w977 -> [_ w1004]
                  tunnel: w985 -> [_ w1003]
                  frame False {
                    n569 = local read "Re-Calculated Values Cluster"() -> (w991:T9)
                    n570 = Unbundle By Name(w991) -> ("Off Current"=w990:dbl)
                    n571 = Divide(x=w995, y=3) -> (x/y=w997:dbl)
                    n572 = Format Value(format string="%#g", value (0)=w990) -> (output string=w992:string)  [unwired: 1 in]
                    n573 = To Word Integer(number=w997) -> (16bit integer=w996:i16)
                    n574 = Replace Array Subset(array=w998, new element=w992, index (row)=w996, index (col)=1) -> (w994:string[][])
                  }
                  frame True {
                    n575 = local read "Re-Calculated Values Cluster"() -> (w1002:T9)
                    n576 = Unbundle By Name(w1002) -> ("Off Current"=w1001:dbl)
                    n577 = Search 1D Array(1D array=w1004, element="On/Off I-Sat:") -> (index of element=w1011:i32)  [unwired: 1 in]
                    n578 = Divide(x=w1011, y=3) -> (x/y=w1012:dbl)
                    n579 = To Word Integer(number=w1012) -> (16bit integer=w1010:i16)
                    n580 = Format Value(format string="%#g", value (0)=w1001) -> (output string=w1015:string)  [unwired: 1 in]
                    n581 = Build Array(w1003, w1015) -> (w1008:string[])
                    n582 = Increment(x=w1010) -> (x+1=w1009:i16)
                    n583 = Insert Into Array(array=w1006, index (row)=w1009, new element=w1008) -> (w1005:string[][])  [unwired: 1 in]
                  }
                }
                n584 = local write "Save Array"(w986) -> ()
              }
              frame #9 {
                w1017 = "Vt-Sat (V):"
                n585 = local read "Save Array"() -> (w1018:string[][])
                n586 = Array Size(array=w1018) -> (size(s)=w1023:i32[])
                n587 = Array Subset(array=w1018, index (row)=0, index (col)=0, length (col)=3) -> (w1019:string[][])  [unwired: 1 in]
                n588 = Index Array(array=w1023, index=0) -> (element=w1025:i32)
                n589 = Reshape Array(w1019, w1025) -> (w1016:string[])
                n590 = Search 1D Array(1D array=w1016, element=w1017) -> (index of element=w1028:i32)  [unwired: 1 in]
                n591 = Equal?(x=w1028, y=-1) -> (x = y?=w1027:bool)
                n592 = case shown="False" w1027 {
                  tunnel: w1018 -> [w1037 w1047]
                  tunnel: w1028 -> [w1033 _]
                  tunnel: [w1032 w1046] -> w1026
                  tunnel: w1017 -> [_ w1045]
                  tunnel: w1016 -> [_ w1044]
                  frame False {
                    n593 = local read "Re-Calculated Values Cluster"() -> (w1031:T9)
                    n594 = Unbundle By Name(w1031) -> ("Vt-Sat"=w1030:dbl)
                    n595 = Divide(x=w1033, y=3) -> (x/y=w1036:dbl)
                    n596 = To Word Integer(number=w1036) -> (16bit integer=w1035:i16)
                    n597 = Number To Fractional String(number=w1030) -> (F-format string=w1034:string)  [unwired: 3 in]
                    n598 = Replace Array Subset(array=w1037, new element=w1034, index (row)=w1035, index (col)=1) -> (w1032:string[][])
                  }
                  frame True {
                    n599 = local read "Re-Calculated Values Cluster"() -> (w1041:T9)
                    n600 = Unbundle By Name(w1041) -> ("Vt-Sat"=w1040:dbl)
                    n601 = Search 1D Array(1D array=w1044, element="Threshold V (V):") -> (index of element=w1043:i32)  [unwired: 1 in]
                    n602 = Divide(x=w1043, y=3) -> (x/y=w1050:dbl)
                    n603 = To Word Integer(number=w1050) -> (16bit integer=w1042:i16)
                    n604 = Format Value(format string="%#g", value (0)=w1040) -> (output string=w1053:string)  [unwired: 1 in]
                    n605 = Build Array(w1045, w1053) -> (w1049:string[])
                    n606 = Replace Array Subset(array=w1047, new element=w1049, index (row)=w1042) -> (w1046:string[][])  [unwired: 1 in]
                  }
                }
                n607 = local write "Save Array"(w1026) -> ()
              }
              frame #10 {
                n608 = disable-structure shown="Disabled" {
                  frame Disabled {
                    n609 = local read "Save Array"() -> (w1054:string[][])
                    n610 = Array Size(array=w1054) -> (size(s)=w1060:i32[])
                    n611 = Array Subset(array=w1054, index (row)=0, index (col)=0, length (col)=3) -> (w1056:string[][])  [unwired: 1 in]
                    n612 = Index Array(array=w1060, index=0) -> (element=w1062:i32)
                    n613 = Reshape Array(w1056, w1062) -> (w1055:string[])
                    n614 = Search 1D Array(1D array=w1055, element="VT-Lin (V):") -> (index of element=w1065:i32)  [unwired: 1 in]
                    n615 = Equal?(x=w1065, y=-1) -> (x = y?=w1064:bool)
                    n616 = case shown="False" w1064 {
                      tunnel: w1054 -> [w1074 w1077]
                      tunnel: w1065 -> [w1071 _]
                      tunnel: [w1070 w1077] -> w1063
                      frame False {
                        n617 = Divide(x=w1071, y=3) -> (x/y=w1073:dbl)
                        n618 = To Word Integer(number=w1073) -> (16bit integer=w1072:i16)
                        n619 = Format Value(format string="%#g") -> (output string=w1068:string)  [unwired: 2 in]
                        n620 = Replace Array Subset(array=w1074, new element=w1068, index (row)=w1072, index (col)=1) -> (w1070:string[][])
                      }
                      frame True {
                      }
                    }
                    n621 = local write "Save Array"(w1063) -> ()
                  }
                  frame Enabled {
                  }
                }
              }
              frame #11 {
                w1078 = "STS-Sat (V/decade):"
                n622 = local read "Save Array"() -> (w1080:string[][])
                n623 = Array Size(array=w1080) -> (size(s)=w1085:i32[])
                n624 = Array Subset(array=w1080, index (row)=0, index (col)=0, length (col)=3) -> (w1081:string[][])  [unwired: 1 in]
                n625 = Index Array(array=w1085, index=0) -> (element=w1087:i32)
                n626 = Reshape Array(w1081, w1087) -> (w1079:string[])
                n627 = Search 1D Array(1D array=w1079, element=w1078) -> (index of element=w1090:i32)  [unwired: 1 in]
                n628 = Equal?(x=w1090, y=-1) -> (x = y?=w1089:bool)
                n629 = case shown="True" w1089 {
                  tunnel: w1080 -> [w1100 w1108]
                  tunnel: w1090 -> [w1097 _]
                  tunnel: [w1096 w1109] -> w1088
                  tunnel: w1079 -> [_ w1107]
                  tunnel: w1078 -> [_ w1106]
                  frame False {
                    n630 = local read "Re-Calculated Values Cluster"() -> (w1092:T9)
                    n631 = Unbundle By Name(w1092) -> ("STS"=w1093:dbl)
                    n632 = Divide(x=w1097, y=3) -> (x/y=w1099:dbl)
                    n633 = To Word Integer(number=w1099) -> (16bit integer=w1098:i16)
                    n634 = Format Value(format string="%#g", value (0)=w1093) -> (output string=w1094:string)  [unwired: 1 in]
                    n635 = Replace Array Subset(array=w1100, new element=w1094, index (row)=w1098, index (col)=1) -> (w1096:string[][])
                  }
                  frame True {
                    n636 = local read "Re-Calculated Values Cluster"() -> (w1103:T9)
                    n637 = Unbundle By Name(w1103) -> ("STS"=w1104:dbl)
                    n638 = Search 1D Array(1D array=w1107, element="S.T.S. (V/decade):") -> (index of element=w1112:i32)  [unwired: 1 in]
                    n639 = Divide(x=w1112, y=3) -> (x/y=w1113:dbl)
                    n640 = To Word Integer(number=w1113) -> (16bit integer=w1105:i16)
                    n641 = Format Value(format string="%#g", value (0)=w1104) -> (output string=w1116:string)  [unwired: 1 in]
                    n642 = Build Array(w1106, w1116) -> (w1111:string[])
                    n643 = Replace Array Subset(array=w1108, new element=w1111, index (row)=w1105) -> (w1109:string[][])  [unwired: 1 in]
                  }
                }
                n644 = local write "Save Array"(w1088) -> ()
              }
              frame #12 {
                w1117 = "Trap Density-VT (Traps/Vcm^2):"
                n645 = local read "Save Array"() -> (w1119:string[][])
                n646 = Array Size(array=w1119) -> (size(s)=w1124:i32[])
                n647 = Array Subset(array=w1119, index (row)=0, index (col)=0, length (col)=3) -> (w1120:string[][])  [unwired: 1 in]
                n648 = Index Array(array=w1124, index=0) -> (element=w1126:i32)
                n649 = Reshape Array(w1120, w1126) -> (w1118:string[])
                n650 = Search 1D Array(1D array=w1118, element=w1117) -> (index of element=w1129:i32)  [unwired: 1 in]
                n651 = Equal?(x=w1129, y=-1) -> (x = y?=w1128:bool)
                n652 = case shown="True" w1128 {
                  tunnel: w1119 -> [w1139 w1146]
                  tunnel: w1129 -> [w1135 _]
                  tunnel: [w1134 w1147] -> w1127
                  tunnel: w1118 -> [_ w1145]
                  tunnel: w1117 -> [_ w1144]
                  frame False {
                    n653 = local read "Re-Calculated Values Cluster"() -> (w1132:T9)
                    n654 = Unbundle By Name(w1132) -> ("Trap Density-VT"=w1131:dbl)
                    n655 = Divide(x=w1135, y=3) -> (x/y=w1138:dbl)
                    n656 = To Word Integer(number=w1138) -> (16bit integer=w1137:i16)
                    n657 = Format Value(format string="%#g", value (0)=w1131) -> (output string=w1136:string)  [unwired: 1 in]
                    n658 = Replace Array Subset(array=w1139, new element=w1136, index (row)=w1137, index (col)=1) -> (w1134:string[][])
                  }
                  frame True {
                    n659 = local read "Re-Calculated Values Cluster"() -> (w1143:T9)
                    n660 = Unbundle By Name(w1143) -> ("Trap Density-VT"=w1142:dbl)
                    n661 = Search 1D Array(1D array=w1145, element="STS-Sat (V/decade):") -> (index of element=w1152:i32)  [unwired: 1 in]
                    n662 = Divide(x=w1152, y=3) -> (x/y=w1151:dbl)
                    n663 = To Word Integer(number=w1151) -> (16bit integer=w1153:i16)
                    n664 = Format Value(format string="%#g", value (0)=w1142) -> (output string=w1148:string)  [unwired: 1 in]
                    n665 = Build Array(w1144, w1148) -> (w1155:string[])
                    n666 = Increment(x=w1153) -> (x+1=w1154:i16)
                    n667 = Insert Into Array(array=w1146, index (row)=w1154, new element=w1155) -> (w1147:string[][])  [unwired: 1 in]
                  }
                }
                n668 = local write "Save Array"(w1127) -> ()
              }
              frame #13 {
                w1157 = "Trap Density-STS (Traps/Vcm^2):"
                n669 = local read "Save Array"() -> (w1159:string[][])
                n670 = Array Size(array=w1159) -> (size(s)=w1164:i32[])
                n671 = Array Subset(array=w1159, index (row)=0, index (col)=0, length (col)=3) -> (w1160:string[][])  [unwired: 1 in]
                n672 = Index Array(array=w1164, index=0) -> (element=w1166:i32)
                n673 = Reshape Array(w1160, w1166) -> (w1158:string[])
                n674 = Search 1D Array(1D array=w1158, element=w1157) -> (index of element=w1169:i32)  [unwired: 1 in]
                n675 = Equal?(x=w1169, y=-1) -> (x = y?=w1168:bool)
                n676 = case shown="True" w1168 {
                  tunnel: w1159 -> [w1179 w1186]
                  tunnel: w1169 -> [w1176 _]
                  tunnel: [w1175 w1187] -> w1167
                  tunnel: w1158 -> [_ w1185]
                  tunnel: w1157 -> [_ w1184]
                  frame False {
                    n677 = local read "Re-Calculated Values Cluster"() -> (w1172:T9)
                    n678 = Unbundle By Name(w1172) -> ("Trap Density-STS"=w1171:dbl)
                    n679 = Divide(x=w1176, y=3) -> (x/y=w1178:dbl)
                    n680 = To Word Integer(number=w1178) -> (16bit integer=w1177:i16)
                    n681 = Format Value(format string="%#g", value (0)=w1171) -> (output string=w1173:string)  [unwired: 1 in]
                    n682 = Replace Array Subset(array=w1179, new element=w1173, index (row)=w1177, index (col)=1) -> (w1175:string[][])
                  }
                  frame True {
                    n683 = local read "Re-Calculated Values Cluster"() -> (w1183:T9)
                    n684 = Unbundle By Name(w1183) -> ("Trap Density-STS"=w1182:dbl)
                    n685 = Search 1D Array(1D array=w1185, element="Trap Density-VT (Traps/Vcm^2):") -> (index of element=w1192:i32)  [unwired: 1 in]
                    n686 = Divide(x=w1192, y=3) -> (x/y=w1193:dbl)
                    n687 = To Word Integer(number=w1193) -> (16bit integer=w1191:i16)
                    n688 = Format Value(format string="%#g", value (0)=w1182) -> (output string=w1196:string)  [unwired: 1 in]
                    n689 = Build Array(w1184, w1196) -> (w1189:string[])
                    n690 = Increment(x=w1191) -> (x+1=w1190:i16)
                    n691 = Insert Into Array(array=w1186, index (row)=w1190, new element=w1189) -> (w1187:string[][])  [unwired: 1 in]
                  }
                }
                n692 = local write "Save Array"(w1167) -> ()
              }
            }
            n693 = local read "New: Temp"() -> (w704:dbl)
            n694 = local read "New: Width"() -> (w705:dbl)
            n695 = local read "New: Length"() -> (w707:dbl)
            n696 = local read "Index"() -> (w706:string)
            n697 = To Single Precision Float(number=w704) -> (single precision float=w721:sgl)
            n698 = Number To Decimal String(number=w721) -> (decimal integer string=w716:string)  [unwired: 1 in]
            n699 = To Single Precision Float(number=w705) -> (single precision float=w720:sgl)
            n700 = To Single Precision Float(number=w707) -> (single precision float=w719:sgl)
            n701 = Strip Path(path=w703) -> (stripped path=w708:path)  [unwired: 1 out]
            n702 = Number To Decimal String(number=w719) -> (decimal integer string=w714:string)  [unwired: 1 in]
            n703 = Number To Decimal String(number=w720) -> (decimal integer string=w713:string)  [unwired: 1 in]
            n704 = Concatenate Strings("_", w716, "K") -> (w718:string)
            n705 = call "Build Text"("Temp"=w718, "Index"=w706, "Length"=w714, "Width"=w713) -> ("Result"=w712:string)  [unwired: 10 in, 1 out]
            n706 = Path To String(path=w708) -> (string=w710:string)
            n707 = Concatenate Strings(w710, "\\", w712) -> (w711:string)
            n708 = String To Path(string=w711) -> (path=w702:path)
          }
          frame #1 {
            n709 = flat-sequence {
              tunnel: w1200 -> [w1202]
              tunnel: w1199 -> [w1201]
              tunnel: [w1201] -> w1198
              tunnel: w1198 -> [w1208]
              tunnel: w1197 -> [w1207]
              frame #0 {
                n710 = Equal?(x=w1202, y=w1201) -> (x = y?=w1203:bool)
                n711 = case shown="False" w1203 {
                  tunnel: w1202 -> [w1206 _]
                  tunnel: w1201 -> [w1205 _]
                  frame False {
                    n712 = Move(source path=w1206, 9:TRUE, 10:w1205) -> ()  [unwired: 2 in, 3 out]
                  }
                  frame True {
                  }
                }
              }
              frame #1 {
                n713 = local write "Transfer File"(w1208) -> ()
                n714 = call-poly <vilib>:"Write To Spreadsheet File.vi"("2D data"=w1207, "file path (dialog if empty)"=w1208) -> ()  [unwired: 6 in, 1 out]
              }
            }
          }
        }
        n715 = Cluster To Array(cluster=w692) -> (array=w691:bool[])
        n716 = Boolean Array To Number(Boolean array=w691) -> (number=w690:u32)
        n717 = Equal To 0?(x=w690) -> (x = 0?=w689:bool)
        n718 = case shown="True" w689 {
          tunnel: [MegaAwesome_States."Read Data" w696] -> w688
          tunnel: w687 -> [_ w700]
          frame False {
          }
          frame True {
            n719 = Unbundle By Name(w700) -> ("Save Next"=w699:bool)
            n720 = Select(t=MegaAwesome_States."No Event", s=w699, f=MegaAwesome_States."Next File") -> (s? t:f=w696:T2)
          }
        }
      }
      frame "Exit" {
      }
      frame "Save Lines" {
        n721 = Build Path(base path=w1213, name or relative path="ROI") -> (appended path=w1216:path)
        n722 = call <vilib>:"Check if File or Folder Exists.vi"("path"=w1216) -> ("file or folder exists?"=w1214:bool, "dup path"=w1217:path)  [unwired: 8 in, 1 out]
        n723 = case shown="False" w1214 {
          tunnel: w1217 -> [w1224 w1225]
          tunnel: [w1223 w1225] -> w1220
          frame False {
            n724 = Create Folder(path (use dialog)=w1224) -> (created path=w1223:path)  [unwired: 2 in, 2 out]
          }
          frame True {
          }
        }
        n725 = local read "Index"() -> (w1212:string)
        n726 = property on="Image Out" class="ImageControl"() -> ("ROI"=w1211:T12)  [unwired: 2 in, 2 out]
        n727 = Build Path(base path=w1220, name or relative path=w1212) -> (appended path=w1219:path)
        n728 = Flatten To String(anything=w1211) -> (data string=w1218:string)  [unwired: 3 in, 2 out]
        n729 = Write to Text File(file (use dialog)=w1219, text=w1218) -> ()  [unwired: 2 in, 3 out]
      }
      frame "Export" {
        n730 = flat-sequence {
          frame #0 {
            n731 = stacked-sequence {
              frame #0 {
                n732 = local read "Independant Variable:"() -> (w1228:string)
                n733 = Equal?(x=w1228, y="Length (um):") -> (x = y?=w1229:bool)
                n734 = case shown="True" w1229 {
                  frame False {
                  }
                  frame True {
                    n735 = local write "X Axis Display Type"("1") -> ()
                    n736 = local write "Opj X Axis"("2") -> ()
                  }
                }
              }
              frame #1 {
                n737 = local read "Independant Variable:"() -> (w1233:string)
                n738 = Equal?(x=w1233, y="Sample Temp (K):") -> (x = y?=w1234:bool)
                n739 = case shown="True" w1234 {
                  frame False {
                  }
                  frame True {
                    n740 = local write "X Axis Display Type"("1") -> ()
                    n741 = local write "Opj X Axis"("1") -> ()
                  }
                }
              }
              frame #2 {
                n742 = local read "Independant Variable:"() -> (w1238:string)
                n743 = Equal?(x=w1238, y="Mobility-Sat (cm^2/Vs):") -> (x = y?=w1239:bool)
                n744 = case shown="True" w1239 {
                  frame False {
                  }
                  frame True {
                    n745 = local write "X Axis Display Type"("2") -> ()
                    n746 = local write "Opj X Axis"("2") -> ()
                  }
                }
              }
              frame #3 {
                n747 = local read "Independant Variable:"() -> (w1243:string)
                n748 = Equal?(x=w1243, y="Mobility-Lin (cm^2/Vs):") -> (x = y?=w1244:bool)
                n749 = case shown="True" w1244 {
                  frame False {
                  }
                  frame True {
                    n750 = local write "X Axis Display Type"("2") -> ()
                    n751 = local write "Opj X Axis"("2") -> ()
                  }
                }
              }
              frame #4 {
                n752 = local read "Independant Variable:"() -> (w1248:string)
                n753 = Equal?(x=w1248, y="On/Off I-Sat:") -> (x = y?=w1249:bool)
                n754 = case shown="True" w1249 {
                  frame False {
                  }
                  frame True {
                    n755 = local write "X Axis Display Type"("2") -> ()
                    n756 = local write "Opj X Axis"("2") -> ()
                  }
                }
              }
              frame #5 {
                n757 = local read "Independant Variable:"() -> (w1253:string)
                n758 = Equal?(x=w1253, y="Off I-Sat (A):") -> (x = y?=w1254:bool)
                n759 = case shown="True" w1254 {
                  frame False {
                  }
                  frame True {
                    n760 = local write "X Axis Display Type"("2") -> ()
                    n761 = local write "Opj X Axis"("2") -> ()
                  }
                }
              }
              frame #6 {
                n762 = local read "Independant Variable:"() -> (w1258:string)
                n763 = Equal?(x=w1258, y="Vt-Sat (V):") -> (x = y?=w1259:bool)
                n764 = case shown="True" w1259 {
                  frame False {
                  }
                  frame True {
                    n765 = local write "X Axis Display Type"("1") -> ()
                    n766 = local write "Opj X Axis"("1") -> ()
                  }
                }
              }
              frame #7 {
                n767 = local read "Independant Variable:"() -> (w1263:string)
                n768 = Equal?(x=w1263, y="STS-Sat (V/decade):") -> (x = y?=w1264:bool)
                n769 = case shown="True" w1264 {
                  frame False {
                  }
                  frame True {
                    n770 = local write "X Axis Display Type"("1") -> ()
                    n771 = local write "Opj X Axis"("1") -> ()
                  }
                }
              }
              frame #8 {
                n772 = local read "Independant Variable:"() -> (w1268:string)
                n773 = Equal?(x=w1268, y="Trap Density-VT (Traps/Vcm^2):") -> (x = y?=w1269:bool)
                n774 = case shown="True" w1269 {
                  frame False {
                  }
                  frame True {
                    n775 = local write "X Axis Display Type"("2") -> ()
                    n776 = local write "Opj X Axis"("2") -> ()
                  }
                }
              }
              frame #9 {
                n777 = local read "Independant Variable:"() -> (w1273:string)
                n778 = Equal?(x=w1273, y="Trap Density-STS (Traps/Vcm^2):") -> (x = y?=w1274:bool)
                n779 = case shown="True" w1274 {
                  frame False {
                  }
                  frame True {
                    n780 = local write "X Axis Display Type"("2") -> ()
                    n781 = local write "Opj X Axis"("2") -> ()
                  }
                }
              }
            }
          }
          frame #1 {
            n782 = local read "Transfer Folder"() -> (w1282:path)
            n783 = Build Path(base path=w1282, name or relative path="Stats") -> (appended path=w1283:path)
            n784 = local read "Origin Project File"() -> (w1294:path)
            n785 = call <vilib>:"Check if File or Folder Exists.vi"("path"=w1283) -> ("file or folder exists?"=w1298:bool, "dup path"=w1297:path)  [unwired: 8 in, 1 out]
            n786 = call <userlib>:"OA_ConnectToOrigin.vi"() -> ("error out"=w1295:errorcluster, "Origin.IOApplication"=w1296:refnum<k7>)  [unwired: 8 in]
            n787 = case shown="False" w1298 {
              tunnel: w1297 -> [w1471 w1472]
              tunnel: [w1470 w1472] -> w1281
              frame False {
                n788 = Create Folder(path (use dialog)=w1471) -> (created path=w1470:path)  [unwired: 2 in, 2 out]
              }
              frame True {
              }
            }
            n789 = call "File Dialog"("start path"=w1283) -> ("selected path"=w1285:path)  [unwired: 11 in, 3 out]
            n790 = call <userlib>:"OA_Load.vi"("error in (no error)"=w1295, "Path"=w1294, "Origin.IOApplication"=w1296) -> ("error out"=w1292:errorcluster, "Origin.IOApplication"=w1293:refnum<k7>)  [unwired: 1 out]
            n791 = call "OAExecute.vi"("script"="document -m 3;", "Error IO"=w1292, "Origin.IOApplication"=w1293) -> ("Error IO Out"=w1290:errorcluster, "Origin.IOApplication"=w1291:refnum<k7>)  [unwired: 1 in, 1 out]
            n792 = local read "Independant Variable:"() -> (w1278:string)
            n793 = stacked-sequence {
              tunnel: w1282 -> [w1309 w1339 w1351 w1373 w1393 w1414 w1435 w1458]
              tunnel: w1281 -> [w1310 w1338 w1352 w1372 w1394 w1415 w1436 w1459]
              tunnel: w1291 -> [w1312 w1336 w1354 w1375 w1396 w1417 w1438 w1461]
              tunnel: w1290 -> [w1311 w1337 w1353 w1374 w1395 w1416 w1437 w1460]
              tunnel: [_ _ _ _ _ _ _ w1456] -> w1280
              tunnel: [_ _ _ _ _ _ _ w1457] -> w1279
              tunnel: w1278 -> [w1308 w1329 w1350 w1371 w1392 w1413 w1434 w1455]
              frame #0 {
                n794 = local read "X Axis Display Type"() -> (w1300:string)
                n795 = local read "Opj X Axis"() -> (w1305:string)
                n796 = Concatenate Strings("window -a MOBLGraph;\nlayer.x.type=", w1305, "; layer.x.label.numFormat = ", w1300, "; Y3 = 1; X3 = 1;", "window -a MOBLTable;\nwindow -s TV;") -> (w1303:string)
                n797 = call "Param_Analysis_7_24b_JW.vi"("Independant Variable"=w1308, "error in (no error)"=w1311, "Data Folder"=w1309, "Parameter String"="Mobility-Lin (cm^2/Vs):", "Parameter Name"="Mobility-Lin", "Stats Folder"=w1310) -> ("error out"=w1314:errorcluster, "Output Array"=w1316:string[][], "Variables"=w1307:T27)  [unwired: 2 in, 1 out]
                n798 = call "Origin_Export_7_27a_JW.vi"("Input Conditions"=w1307, "Analysis Array"=w1316, "error in (no error)"=w1314, "Parameter Worksheet Name"="[MOBLTable]Mobilities", "Parameter Folder Script"="pe_cd \"Mobility-Lin\";", "Origin.IOApplication"=w1312) -> ("error out"=w1313:errorcluster, "reference out"=w1315:refnum<k7>)  [unwired: 3 in, 1 out]
                n799 = call "OAExecute.vi"("script"=w1303, "Error IO"=w1313, "Origin.IOApplication"=w1315) -> ()  [unwired: 1 in, 3 out]
              }
              frame #1 {
                n800 = local read "X Axis Display Type"() -> (w1321:string)
                n801 = local read "Opj X Axis"() -> (w1326:string)
                n802 = Concatenate Strings("window -a MOBSGraph;\nlayer.x.type=", w1326, "; layer.x.label.numFormat = ", w1321, "; Y3 = 1; X3 = 1;", "window -a MOBSTable;\nwindow -s TV;") -> (w1324:string)
                n803 = call "Param_Analysis_7_24b_JW.vi"("Independant Variable"=w1329, "error in (no error)"=w1337, "Data Folder"=w1339, "Parameter String"="Mobility-Sat (cm^2/Vs):", "Parameter Name"="Mobility-Sat", "Stats Folder"=w1338) -> ("error out"=w1332:errorcluster, "Output Array"=w1330:string[][], "Variables"=w1328:T27)  [unwired: 2 in, 1 out]
                n804 = call "Origin_Export_7_27a_JW.vi"("Input Conditions"=w1328, "Analysis Array"=w1330, "error in (no error)"=w1332, "Parameter Worksheet Name"="[MOBSTable]Mobilities", "Parameter Folder Script"="pe_cd \"Mobility-Sat\";", "Origin.IOApplication"=w1336) -> ("error out"=w1331:errorcluster, "reference out"=w1333:refnum<k7>)  [unwired: 3 in, 1 out]
                n805 = call "OAExecute.vi"("script"=w1324, "Error IO"=w1331, "Origin.IOApplication"=w1333) -> ()  [unwired: 1 in, 3 out]
              }
              frame #2 {
                n806 = local read "X Axis Display Type"() -> (w1342:string)
                n807 = local read "Opj X Axis"() -> (w1347:string)
                n808 = Concatenate Strings("window -a NSTSGraph;\nlayer.x.type=", w1347, "; layer.x.label.numFormat = ", w1342, "; Y3 = 1; X3 = 1;", "window -a NSTSTable;\nwindow -s TV;") -> (w1345:string)
                n809 = call "Param_Analysis_7_24b_JW.vi"("Independant Variable"=w1350, "error in (no error)"=w1353, "Data Folder"=w1351, "Parameter String"="Trap Density-STS (Traps/Vcm^2):", "Parameter Name"="Trap Density-STS", "Stats Folder"=w1352) -> ("error out"=w1357:errorcluster, "Output Array"=w1355:string[][], "Variables"=w1349:T27)  [unwired: 2 in, 1 out]
                n810 = call "Origin_Export_7_27a_JW.vi"("Input Conditions"=w1349, "Analysis Array"=w1355, "error in (no error)"=w1357, "Parameter Worksheet Name"="[NSTSTable]Trap Densities", "Parameter Folder Script"="pe_cd \"N-STS\";", "Origin.IOApplication"=w1354) -> ("error out"=w1356:errorcluster, "reference out"=w1358:refnum<k7>)  [unwired: 3 in, 1 out]
                n811 = call "OAExecute.vi"("script"=w1345, "Error IO"=w1356, "Origin.IOApplication"=w1358) -> ()  [unwired: 1 in, 3 out]
              }
              frame #3 {
                n812 = local read "X Axis Display Type"() -> (w1363:string)
                n813 = local read "Opj X Axis"() -> (w1368:string)
                n814 = call "Param_Analysis_7_24b_JW.vi"("Independant Variable"=w1371, "error in (no error)"=w1374, "Data Folder"=w1373, "Parameter String"="Trap Density-VT (Traps/Vcm^2):", "Parameter Name"="Trap Density-Vt", "Stats Folder"=w1372) -> ("error out"=w1378:errorcluster, "Output Array"=w1376:string[][], "Variables"=w1370:T27)  [unwired: 2 in, 1 out]
                n815 = Concatenate Strings("window -a NVtGraph;\nlayer.x.type=", w1368, "; layer.x.label.numFormat = ", w1363, "; Y3 = 1; X3 = 1;", "window -a NVtTable;\nwindow -s TV;") -> (w1366:string)
                n816 = call "Origin_Export_7_27a_JW.vi"("Input Conditions"=w1370, "Analysis Array"=w1376, "error in (no error)"=w1378, "Parameter Worksheet Name"="[NVTTable]Trap Densities", "Parameter Folder Script"="pe_cd \"N-Vt\";", "Origin.IOApplication"=w1375) -> ("error out"=w1377:errorcluster, "reference out"=w1379:refnum<k7>)  [unwired: 3 in, 1 out]
                n817 = call "OAExecute.vi"("script"=w1366, "Error IO"=w1377, "Origin.IOApplication"=w1379) -> ()  [unwired: 1 in, 3 out]
              }
              frame #4 {
                n818 = local read "X Axis Display Type"() -> (w1384:string)
                n819 = local read "Opj X Axis"() -> (w1389:string)
                n820 = Concatenate Strings("window -a OffIGraph;\nlayer.x.type=", w1389, "; layer.x.label.numFormat = ", w1384, "; Y3 = 1; X3 = 1;", "window -a OffITable;\nwindow -s TV;") -> (w1387:string)
                n821 = call "Param_Analysis_7_24b_JW.vi"("Independant Variable"=w1392, "error in (no error)"=w1395, "Data Folder"=w1393, "Parameter String"="Off I-Sat (A):", "Parameter Name"="Off I-Sat", "Stats Folder"=w1394) -> ("error out"=w1399:errorcluster, "Output Array"=w1397:string[][], "Variables"=w1391:T27)  [unwired: 2 in, 1 out]
                n822 = call "Origin_Export_7_27a_JW.vi"("Input Conditions"=w1391, "Analysis Array"=w1397, "error in (no error)"=w1399, "Parameter Worksheet Name"="[OffItable]OffCurrents", "Parameter Folder Script"="pe_cd \"OffI-Sat\";", "Origin.IOApplication"=w1396) -> ("error out"=w1398:errorcluster, "reference out"=w1400:refnum<k7>)  [unwired: 3 in, 1 out]
                n823 = call "OAExecute.vi"("script"=w1387, "Error IO"=w1398, "Origin.IOApplication"=w1400) -> ()  [unwired: 1 in, 3 out]
              }
              frame #5 {
                n824 = local read "X Axis Display Type"() -> (w1405:string)
                n825 = local read "Opj X Axis"() -> (w1410:string)
                n826 = Concatenate Strings("window -a OnOffGraph;\nlayer.x.type=", w1410, "; layer.x.label.numFormat = ", w1405, "; Y3 = 1; X3 = 1;", "window -a OnOffTable;\nwindow -s TV;") -> (w1408:string)
                n827 = call "Param_Analysis_7_24b_JW.vi"("Independant Variable"=w1413, "error in (no error)"=w1416, "Data Folder"=w1414, "Parameter String"="On/Off I-Sat:", "Parameter Name"="OnOff Ratio", "Stats Folder"=w1415) -> ("error out"=w1420:errorcluster, "Output Array"=w1418:string[][], "Variables"=w1412:T27)  [unwired: 2 in, 1 out]
                n828 = call "Origin_Export_7_27a_JW.vi"("Input Conditions"=w1412, "Analysis Array"=w1418, "error in (no error)"=w1420, "Parameter Worksheet Name"="[OnOffTable]On/Off Ratios", "Parameter Folder Script"="pe_cd \"OnOff-Ratio\";", "Origin.IOApplication"=w1417) -> ("error out"=w1419:errorcluster, "reference out"=w1421:refnum<k7>)  [unwired: 3 in, 1 out]
                n829 = call "OAExecute.vi"("script"=w1408, "Error IO"=w1419, "Origin.IOApplication"=w1421) -> ()  [unwired: 1 in, 3 out]
              }
              frame #6 {
                n830 = local read "X Axis Display Type"() -> (w1426:string)
                n831 = local read "Opj X Axis"() -> (w1431:string)
                n832 = call "Param_Analysis_7_24b_JW.vi"("Independant Variable"=w1434, "error in (no error)"=w1437, "Data Folder"=w1435, "Parameter String"="STS-Sat (V/decade):", "Parameter Name"="STS-Sat", "Stats Folder"=w1436) -> ("error out"=w1441:errorcluster, "Output Array"=w1439:string[][], "Variables"=w1433:T27)  [unwired: 2 in, 1 out]
                n833 = Concatenate Strings("window -a SGraph;\nlayer.x.type=", w1431, "; layer.x.label.numFormat = ", w1426, "; Y3 = 1; X3 = 1;", "window -a STable;\nwindow -s TV;") -> (w1429:string)
                n834 = call "Origin_Export_7_27a_JW.vi"("Input Conditions"=w1433, "Analysis Array"=w1439, "error in (no error)"=w1441, "Parameter Worksheet Name"="[STable]Threshold Swing", "Parameter Folder Script"="pe_cd \"STS-Sat\";", "Origin.IOApplication"=w1438) -> ("error out"=w1440:errorcluster, "reference out"=w1442:refnum<k7>)  [unwired: 3 in, 1 out]
                n835 = call "OAExecute.vi"("script"=w1429, "Error IO"=w1440, "Origin.IOApplication"=w1442) -> ()  [unwired: 1 in, 3 out]
              }
              frame #7 {
                n836 = local read "X Axis Display Type"() -> (w1447:string)
                n837 = local read "Opj X Axis"() -> (w1452:string)
                n838 = Concatenate Strings("window -a VtGraph;\nlayer.x.type=", w1452, "; layer.x.label.numFormat = ", w1447, "; Y3 = 1; X3 = 1;", "window -a VtTable;\nwindow -s TV;") -> (w1450:string)
                n839 = call "Param_Analysis_7_24b_JW.vi"("Independant Variable"=w1455, "error in (no error)"=w1460, "Data Folder"=w1458, "Parameter String"="Vt-Sat (V):", "Parameter Name"="Vt-Sat", "Stats Folder"=w1459) -> ("error out"=w1464:errorcluster, "Output Array"=w1462:string[][], "Variables"=w1454:T27)  [unwired: 2 in, 1 out]
                n840 = call "Origin_Export_7_27a_JW.vi"("Input Conditions"=w1454, "Analysis Array"=w1462, "error in (no error)"=w1464, "Parameter Worksheet Name"="[VtTable]Threshold Voltages", "Parameter Folder Script"="pe_cd \"Vt-Sat\";", "Origin.IOApplication"=w1461) -> ("error out"=w1463:errorcluster, "reference out"=w1465:refnum<k7>)  [unwired: 3 in, 1 out]
                n841 = call "OAExecute.vi"("script"=w1450, "Error IO"=w1463, "Origin.IOApplication"=w1465) -> ("Error IO Out"=w1456:errorcluster, "Origin.IOApplication"=w1457:refnum<k7>)  [unwired: 1 in, 1 out]
              }
            }
            n842 = Path To String(path=w1285) -> (string=w1284:string)
            n843 = call "OAExecute.vi"("script"="pe_cd /; ", "Error IO"=w1280, "Origin.IOApplication"=w1279) -> ("Error IO Out"=w1286:errorcluster, "Origin.IOApplication"=w1287:refnum<k7>)  [unwired: 1 in, 1 out]
            n844 = call <userlib>:"OASaveProject.vi"("path"=w1284, "Error IO"=w1286, "Origin.IOApplication"=w1287) -> ()  [unwired: 3 out]
          }
        }
      }
    }
    "Current State" <- w16
    "Folder Index" <- w9
    n845 = Equal?(x=w18, y=MegaAwesome_States."Exit") -> (x = y?=w19:bool)
    n846 = Select(t=50, s="Include Images?", f=5) -> (s? t:f=w5:i32)
    n847 = Wait (ms)(milliseconds to wait=w5) -> ()  [unwired: 1 out]
  }
